vi "3 Phase Generator PMU Testing.vi"() -> ()   [LabVIEW 2022 SP3]
uses:
  <vilib>/Utility/TDMS File Viewer/NI_TDMS File Viewer.lvlib
  <vilib>/measure/NI_MAPro.lvlib
  <vilib>/Waveform/WDTOps.llb/WDT Get Waveform Time Array DBL.vi
  <vilib>/measure/maresamp.llb/Align 1 + N Waveforms (continuous).vi
panel:
  out "Phase 2":picture caption="Phasors visualization"
  in  "Data type":i32=8
  in  "ROCOF":dbl caption="Offset"
  in  "Data save 2":bool
  in  "Data save":bool
  in  "?":enum32{"Test set-up", "Set up"}(tab)
  out "h2rad":string="rad"
  out "h1rad":string="rad"
  out "h2deg\nH2deg":string="deg"
  out "H1deg":string="deg"
  out "H2V":string="V"
  out "H1V":string="V"
  out "H2pu":string="pu"
  out "H1pu":string="pu"
  out "PMrad":string="rad"
  out "PMdeg":string="deg"
  out "PMFeq":string="Hz"
  out "FreqDev":string="Hz"
  out "second":string="s"
  out "Hz/s":string="Hz/s"
  out "Final freq":string="Hz"
  out "Voltage step (V)":string="V"
  out "Voltage step (pu)":string="pu"
  out "?":string="Hz"
  out "AM (V)":string="V"
  out "AM (pu)":string="pu"
  out "?":string="Hz"
  out "?":string="Hz"
  out "?":string="V"
  out "?":string="pu"
  in  "H2 order":dbl=5.0 format="%#_13g"
  in  "Start":bool
  in  "Final freq.":dbl=55.0 format="%.2f"
  in  "ROCOF rate":dbl=1.0 format="%.2f"
  in  "Select test type":u16(ring) items=["Steady state", "Voltage step", "Phase step", "Frequency step", "Frequency ramp", "Amplitude modulation", "Phase modulation", "Harmonics"]
  in  "Frequency step":dbl caption="Offset" min=-5.0 max=5.0 format="%#.6f"
  in  "Phase step":dbl caption="Offset" min=-360.0 max=360.0 format="%#.6f"
  in  "Phase":dbl caption="Offset" min=-360.0 max=360.0
  in  "Voltage":dbl=1.0 caption="Offset" max=1.25 format="%#_5g"
  in  "Voltage step":dbl caption="Offset" min=-0.25 max=0.25 format="%#.6f"
  in  "Frequency":dbl=50.0 caption="Offset" max=55.0 format="%#_7g"
  in  "Mod Freq":dbl=1.0 caption="Offset" min=0.0 max=2.384 step=0.1 format="%#.6f"
  in  "Mod Amp":dbl=0.1 caption="Offset" max=0.125 format="%#.4f"
  in  "Mod Amp":dbl=0.1 caption="Offset" max=15.0 format="%#.4f"
  in  "Mod Freq":dbl=1.0 caption="Offset" format="%#.6f"
  in  "Nominal voltage":dbl=230.0 caption="Offset" format="%_6f"
  in  "stop":bool
  in  "Phase":dbl caption="Offset"
  in  "H1 Volt":dbl=0.05 format="%#_13g"
  in  "H2 Volt":dbl=0.05 format="%#_13g"
  in  "H1 Phase":dbl format="%#_13g"
  in  "H1 order":dbl=3.0 format="%#_13g"
  in  "H2 Phase":dbl format="%#_13g"
  out "Freq Dev":dbl caption="Offset" max=15.0 format="%#.4f"
  out "ROCOF":dbl
  out "Frequency":dbl=50.0 format="%#.8g"
  out "Voltage":dbl=1.0 format="%#_7g"
  out "Phase":dbl
  out "Phase (rad)":string="rad"
  out "Phase (deg)":string="deg"
  out "Time":dbl
  in  "File Name":string="testfile.tdms" caption="File name"
  in  "start":bool
  out "Phase step (rad)":string="rad"
  out "Phase step (deg)":string="deg"
  in  "Nominal Voltage":dbl=230.0 format="%#_13g"
  out "Transmitted Data":string
  in  "Voltage unit":u16(ring)=1 items=["Nominal voltage", "Per-unit voltage"]
  in  "Phase unit":u16(ring) items=["Degree", "Radian"]
  in  "Sampling info":cluster{"Fs":dbl, "#s":dbl}={"Fs"=10000.0, "#s"=1000.0} {"Fs" format="%.2p"}
  in  "LAN Module IP Address":string
  in  "LAN Port":u16
  in  "Nominal Frequency":dbl=50.0 format="%#_13g"
  out "Phase waveform 2":dbl(graph)
  in  "Initial freq.":dbl=50.0 format="%.2f"
  out "ROCOF waveform 2":dbl(graph)
  out "ROCOF waveform":dynamicdata(graph)
  out "Frequency waveform 2":dbl(graph)
  out "Frequency waveform":dynamicdata(graph)
  out "Votlage waveform":dynamicdata(graph)
  out "Numeric":i32
  out "resulting string 2":string
  out "double precision float":dbl[](array[numeric])
  out "Array 3":dbl[](array[numeric])
  out "Array 2":dbl[](array[numeric])
  out "Array":dbl[](array[numeric])
  out "Phase waveform":waveform(dbl)(graph)
  # "Current phasor values"
  # "UDP Protocol"
  # "Waveform scaling"
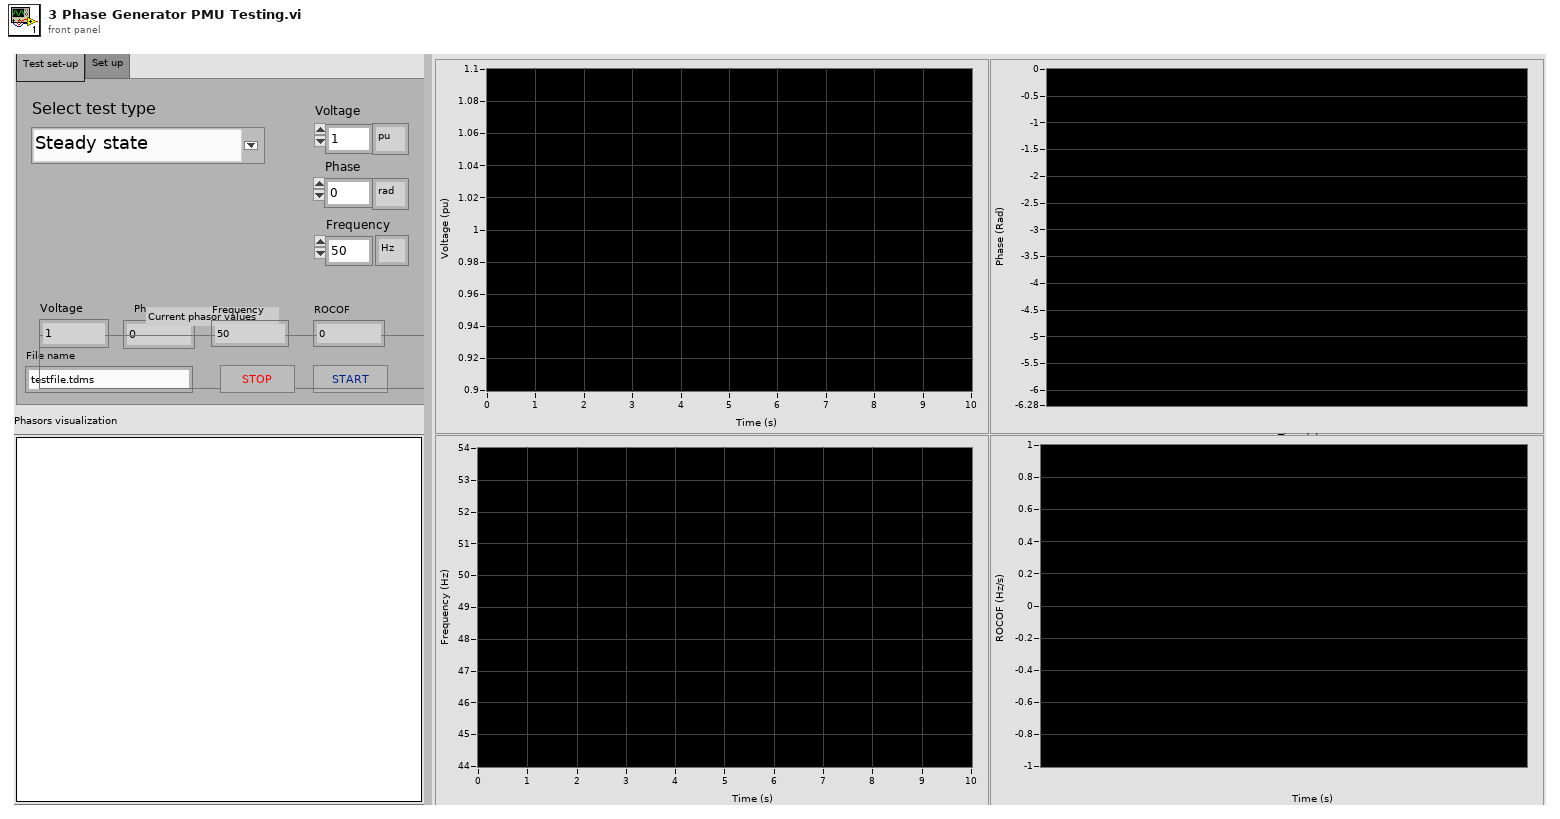
[diagram p1: front panel]
types:
  T1 = enum16{"open", "open or create", "create or replace", "create", "open (read-only)"}
  T2 = cluster{"maximum":dbl, "minimum":dbl, "clip to min":bool, "log?(F)":bool, "grid color":u32, "plot color":u32, "fmt and prec":cluster{"format":enum8{"Decimal", "Scientific", "Engineering", "Binary", "Octal", "Hex"}, "precision":u8}, "visible section":u16}
  T3 = typedef "LVBoundsTypeDef.ctl" = cluster{"Width":u32, "Height":u32}
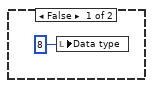
[diagram p2: hidden frame]
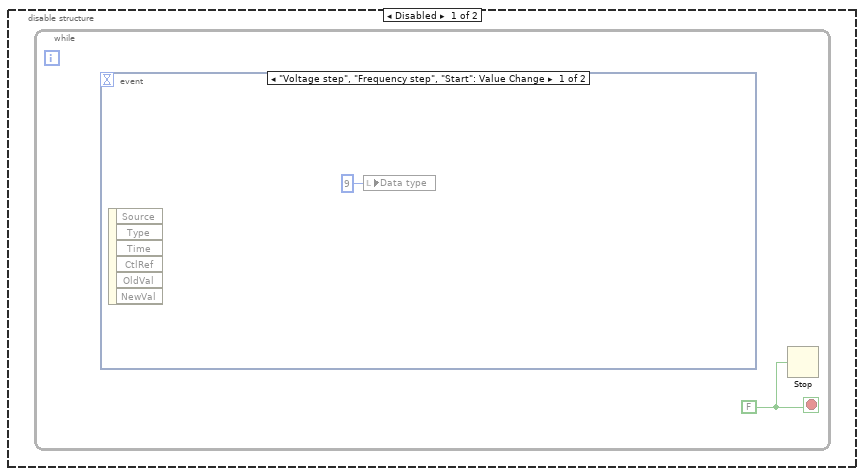
[diagram p3: hidden frame]
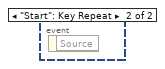
[diagram p4: hidden frame]
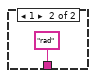
[diagram p5: hidden frame]
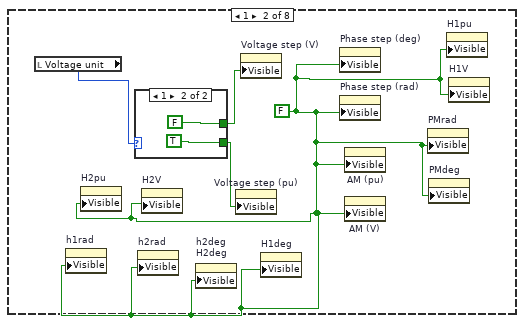
[diagram p6: hidden frame]
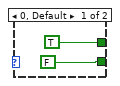
[diagram p7: hidden frame]
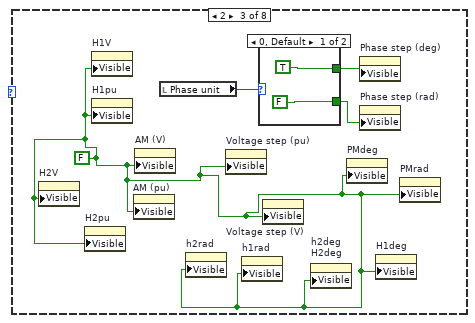
[diagram p8: hidden frame]
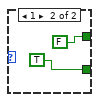
[diagram p9: hidden frame]
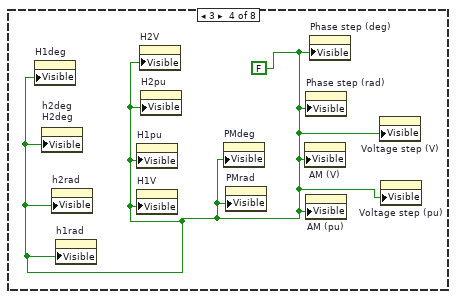
[diagram p10: hidden frame]
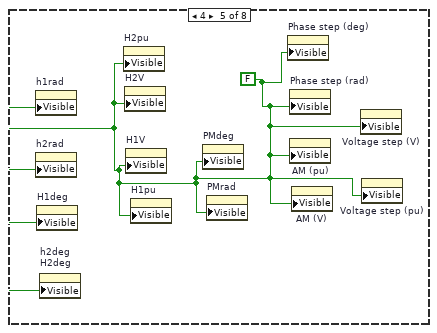
[diagram p11: hidden frame]
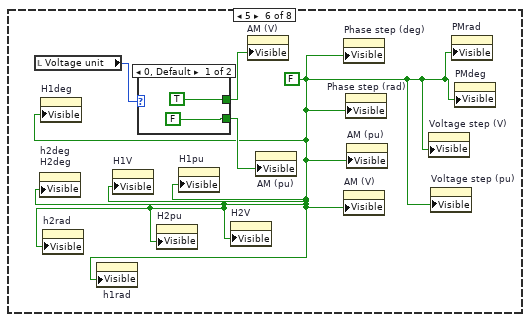
[diagram p12: hidden frame]
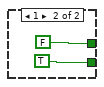
[diagram p13: hidden frame]
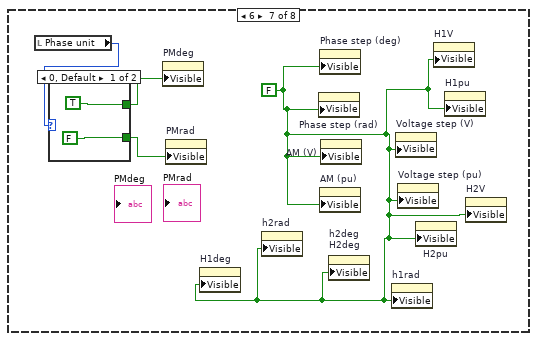
[diagram p14: hidden frame]
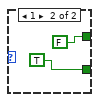
[diagram p15: hidden frame]
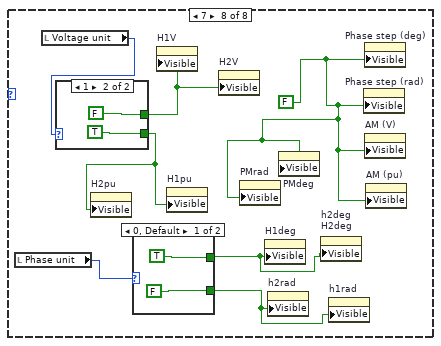
[diagram p16: hidden frame]
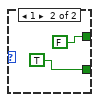
[diagram p17: hidden frame]
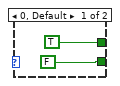
[diagram p18: hidden frame]
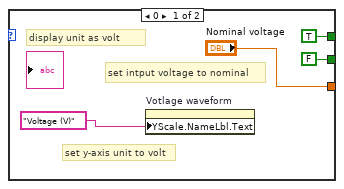
[diagram p19: hidden frame]
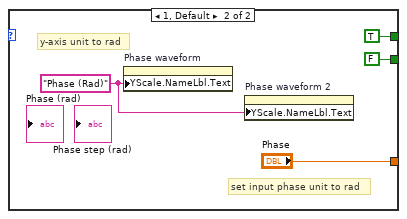
[diagram p20: hidden frame]
diagram:
  n1 = call <vilib>:"Application Directory.vi"() -> ("Application Directory"=w5:path)
  n2 = Concatenate Strings("measurements\\", "File Name") -> (w3:string)
  n3 = Build Path(base path=w5, name or relative path=w3) -> (appended path=w4:path)
  n4 = flat-sequence {
    frame #0 {
      w23 = FALSE
      n5 = local read "Data type"() -> (w29:i32)
      n6 = local read "start"() -> (w22:bool)
      n7 = Equal?(x=w29, y=8) -> (x = y?=w28:bool)
      n8 = Equal?(x=w22, y=TRUE) -> (x = y?=w27:bool)
      n9 = And(x=w27, y=w28) -> (x .and. y?=w26:bool)
      n10 = case shown="True" w26 {
        frame False {
          n11 = local write "Data type"(8 ("Data type")) -> ()
        }
        frame True {
          n12 = local write "Data type"(9 ("Data type")) -> ()
        }
      }
      n13 = property on="Start" class="Bool (strict)"("Value"=w23) -> ()  [unwired: 2 in, 2 out]
      n14 = property on="start" class="Bool (strict)"("Value"=w23) -> ()  [unwired: 2 in, 2 out]
    }
  }
  n15 = TDMS Open(10:T1."create or replace" ("operation (0:open)"), 11:w4) -> (0:w14:errorcluster, 3:w15:refnum<k34>)  [unwired: 5 in]
  n16 = TDMS Set Properties(5:"Data file for PMU testing", 7:"title", 8:w14, 11:w15) -> (0:w12:errorcluster, 3:w13:refnum<k34>)  [unwired: 2 in, 2 out]
  n17 = Get Date/Time In Seconds() -> (seconds since 1Jan1904=w16:timestamp)
  n18 = TDMS Set Properties(5:w16, 7:"datetime", 8:w12, 11:w13) -> (0:w7:errorcluster, 3:w6:refnum<k34>)  [unwired: 2 in, 2 out]
  n19 = while {
    tunnel: [w37] -> w18
    tunnel: [w36] -> w17
    tunnel: w7 -> [w34]
    tunnel: w6 -> [w35]
    i -> [w69]
    stop <- "stop" stop-if-true
    w44 = "3 Phase Generator" ("group name in (Untitled)")
    # "amplitude modulation\nmod freq unit"
    # "phase \nmodulation\namplitude \nunit"
    # "stop button"
    # "box for config layout"
    n20 = flat-sequence {
      tunnel: ["start"] -> w40
      tunnel: ["start"] -> _
      tunnel: [w87] -> w43
      tunnel: [w82] -> w42
      tunnel: [w85] -> w41
      tunnel: w40 -> [w87]
      tunnel: [w166] -> w74
      tunnel: w43 -> [w166]
      tunnel: w42 -> [w160]
      tunnel: w41 -> [w178]
      tunnel: w39 -> [w174]
      tunnel: w38 -> [w173]
      tunnel: [w172] -> w37
      tunnel: [w171] -> w36
      tunnel: w74 -> [w790]
      frame #0 {
        # "input freq unit"
        # "start button"
      }
      frame #1 {
        # "voltage step"
        # "amplitude modulation unit"
        # "set default angle unit ot rad\nif input deg, convert to rad"
        # "enable nominal voltage"
        # "enable unit volt"
        # "enable unit per-unit"
        # "enable per-unit voltage"
        # "per-unit voltage or nominal voltage"
        n21 = local read "Select test type"() -> (w80:u16)
        n22 = case shown="0" "Phase unit" {
          tunnel: [w147 "Phase"] -> w82
          tunnel: [FALSE TRUE] -> w78
          tunnel: [TRUE FALSE] -> w79
          frame 0 {
            # "convert deg to rad"
            # "y-axis in deg"
            # "set inputphase unit to deg"
            n23 = property on="Phase waveform" class="WFChart (strict)"("YScale.NameLbl.Text"="Phase (deg)" ("Y Scale.Name Label.Text")) -> ()  [unwired: 2 in, 2 out]
            n24 = Multiply(x="Phase", y=3.141592653589793) -> (x*y=w150:dbl)
            n25 = Divide(x=w150, y=180.0) -> (x/y=w147:dbl)
          }
          frame 1, Default {
            w154 = "Phase (Rad)" ("Y Scale.Name Label.Text")
            # "y-axis unit to rad"
            # "set input phase unit to rad"
            n26 = property on="Phase waveform" class="WFChart (strict)"("YScale.NameLbl.Text"=w154) -> ()  [unwired: 2 in, 2 out]
            n27 = property on="Phase waveform 2" class="WFChart (strict)"("YScale.NameLbl.Text"=w154) -> ()  [unwired: 2 in, 2 out]
          }
        }
        n28 = case shown="0, Default" w80 {
          frame 0, Default {
            w88 = FALSE
            n29 = property on="H2V" class="Str"("Visible"=w88) -> ()  [unwired: 2 in, 2 out]
            n30 = property on="H2pu" class="Str"("Visible"=w88) -> ()  [unwired: 2 in, 2 out]
            n31 = property on="h1rad" class="Str"("Visible"=w88) -> ()  [unwired: 2 in, 2 out]
            n32 = property on="H1deg" class="Str"("Visible"=w88) -> ()  [unwired: 2 in, 2 out]
            n33 = property on="H1V" class="Str"("Visible"=w88) -> ()  [unwired: 2 in, 2 out]
            n34 = property on="H1pu" class="Str"("Visible"=w88) -> ()  [unwired: 2 in, 2 out]
            n35 = property on="h2rad" class="Str"("Visible"=w88) -> ()  [unwired: 2 in, 2 out]
            n36 = property on="h2deg\nH2deg" class="Str"("Visible"=w88) -> ()  [unwired: 2 in, 2 out]
            n37 = property on="PMdeg" class="Str"("Visible"=w88) -> ()  [unwired: 2 in, 2 out]
            n38 = property on="PMrad" class="Str"("Visible"=w88) -> ()  [unwired: 2 in, 2 out]
            n39 = property on="Voltage step (pu)" class="Str"("Visible"=w88) -> ()  [unwired: 2 in, 2 out]
            n40 = property on="AM (pu)" class="Str"("Visible"=w88) -> ()  [unwired: 2 in, 2 out]
            n41 = property on="AM (V)" class="Str"("Visible"=w88) -> ()  [unwired: 2 in, 2 out]
            n42 = property on="Phase step (deg)" class="Str"("Visible"=w88) -> ()  [unwired: 2 in, 2 out]
            n43 = property on="Phase step (rad)" class="Str"("Visible"=w88) -> ()  [unwired: 2 in, 2 out]
            n44 = property on="Voltage step (V)" class="Str"("Visible"=w88) -> ()  [unwired: 2 in, 2 out]
          }
          frame 1 {
            w89 = FALSE
            n45 = local read "Voltage unit"() -> (w92:u16)
            n46 = property on="h1rad" class="Str"("Visible"=w89) -> ()  [unwired: 2 in, 2 out]
            n47 = property on="H2pu" class="Str"("Visible"=w89) -> ()  [unwired: 2 in, 2 out]
            n48 = case shown="1" w92 {
              tunnel: [TRUE FALSE] -> w90
              tunnel: [FALSE TRUE] -> w91
              frame 0, Default {
              }
              frame 1 {
              }
            }
            n49 = property on="h2rad" class="Str"("Visible"=w89) -> ()  [unwired: 2 in, 2 out]
            n50 = property on="H2V" class="Str"("Visible"=w89) -> ()  [unwired: 2 in, 2 out]
            n51 = property on="h2deg\nH2deg" class="Str"("Visible"=w89) -> ()  [unwired: 2 in, 2 out]
            n52 = property on="Voltage step (pu)" class="Str"("Visible"=w91) -> ()  [unwired: 2 in, 2 out]
            n53 = property on="Voltage step (V)" class="Str"("Visible"=w90) -> ()  [unwired: 2 in, 2 out]
            n54 = property on="H1deg" class="Str"("Visible"=w89) -> ()  [unwired: 2 in, 2 out]
            n55 = property on="Phase step (deg)" class="Str"("Visible"=w89) -> ()  [unwired: 2 in, 2 out]
            n56 = property on="Phase step (rad)" class="Str"("Visible"=w89) -> ()  [unwired: 2 in, 2 out]
            n57 = property on="AM (pu)" class="Str"("Visible"=w89) -> ()  [unwired: 2 in, 2 out]
            n58 = property on="AM (V)" class="Str"("Visible"=w89) -> ()  [unwired: 2 in, 2 out]
            n59 = property on="PMrad" class="Str"("Visible"=w89) -> ()  [unwired: 2 in, 2 out]
            n60 = property on="PMdeg" class="Str"("Visible"=w89) -> ()  [unwired: 2 in, 2 out]
            n61 = property on="H1pu" class="Str"("Visible"=w89) -> ()  [unwired: 2 in, 2 out]
            n62 = property on="H1V" class="Str"("Visible"=w89) -> ()  [unwired: 2 in, 2 out]
          }
          frame 2 {
            w97 = FALSE
            n63 = property on="H2V" class="Str"("Visible"=w97) -> ()  [unwired: 2 in, 2 out]
            n64 = property on="H2pu" class="Str"("Visible"=w97) -> ()  [unwired: 2 in, 2 out]
            n65 = property on="H1V" class="Str"("Visible"=w97) -> ()  [unwired: 2 in, 2 out]
            n66 = property on="H1pu" class="Str"("Visible"=w97) -> ()  [unwired: 2 in, 2 out]
            n67 = property on="AM (pu)" class="Str"("Visible"=w97) -> ()  [unwired: 2 in, 2 out]
            n68 = property on="AM (V)" class="Str"("Visible"=w97) -> ()  [unwired: 2 in, 2 out]
            n69 = local read "Phase unit"() -> (w98:u16)
            n70 = property on="h2rad" class="Str"("Visible"=w97) -> ()  [unwired: 2 in, 2 out]
            n71 = property on="Voltage step (pu)" class="Str"("Visible"=w97) -> ()  [unwired: 2 in, 2 out]
            n72 = property on="h1rad" class="Str"("Visible"=w97) -> ()  [unwired: 2 in, 2 out]
            n73 = case shown="0, Default" w98 {
              tunnel: [TRUE FALSE] -> w100
              tunnel: [FALSE TRUE] -> w99
              frame 0, Default {
              }
              frame 1 {
              }
            }
            n74 = property on="Voltage step (V)" class="Str"("Visible"=w97) -> ()  [unwired: 2 in, 2 out]
            n75 = property on="h2deg\nH2deg" class="Str"("Visible"=w97) -> ()  [unwired: 2 in, 2 out]
            n76 = property on="PMdeg" class="Str"("Visible"=w97) -> ()  [unwired: 2 in, 2 out]
            n77 = property on="Phase step (deg)" class="Str"("Visible"=w100) -> ()  [unwired: 2 in, 2 out]
            n78 = property on="Phase step (rad)" class="Str"("Visible"=w99) -> ()  [unwired: 2 in, 2 out]
            n79 = property on="H1deg" class="Str"("Visible"=w97) -> ()  [unwired: 2 in, 2 out]
            n80 = property on="PMrad" class="Str"("Visible"=w97) -> ()  [unwired: 2 in, 2 out]
          }
          frame 3 {
            w105 = FALSE
            n81 = property on="H1deg" class="Str"("Visible"=w105) -> ()  [unwired: 2 in, 2 out]
            n82 = property on="h2deg\nH2deg" class="Str"("Visible"=w105) -> ()  [unwired: 2 in, 2 out]
            n83 = property on="h2rad" class="Str"("Visible"=w105) -> ()  [unwired: 2 in, 2 out]
            n84 = property on="h1rad" class="Str"("Visible"=w105) -> ()  [unwired: 2 in, 2 out]
            n85 = property on="H1pu" class="Str"("Visible"=w105) -> ()  [unwired: 2 in, 2 out]
            n86 = property on="H1V" class="Str"("Visible"=w105) -> ()  [unwired: 2 in, 2 out]
            n87 = property on="H2V" class="Str"("Visible"=w105) -> ()  [unwired: 2 in, 2 out]
            n88 = property on="H2pu" class="Str"("Visible"=w105) -> ()  [unwired: 2 in, 2 out]
            n89 = property on="PMdeg" class="Str"("Visible"=w105) -> ()  [unwired: 2 in, 2 out]
            n90 = property on="PMrad" class="Str"("Visible"=w105) -> ()  [unwired: 2 in, 2 out]
            n91 = property on="AM (V)" class="Str"("Visible"=w105) -> ()  [unwired: 2 in, 2 out]
            n92 = property on="Phase step (rad)" class="Str"("Visible"=w105) -> ()  [unwired: 2 in, 2 out]
            n93 = property on="AM (pu)" class="Str"("Visible"=w105) -> ()  [unwired: 2 in, 2 out]
            n94 = property on="Phase step (deg)" class="Str"("Visible"=w105) -> ()  [unwired: 2 in, 2 out]
            n95 = property on="Voltage step (V)" class="Str"("Visible"=w105) -> ()  [unwired: 2 in, 2 out]
            n96 = property on="Voltage step (pu)" class="Str"("Visible"=w105) -> ()  [unwired: 2 in, 2 out]
          }
          frame 4 {
            w106 = FALSE
            n97 = property on="h1rad" class="Str"("Visible"=w106) -> ()  [unwired: 2 in, 2 out]
            n98 = property on="h2rad" class="Str"("Visible"=w106) -> ()  [unwired: 2 in, 2 out]
            n99 = property on="H1deg" class="Str"("Visible"=w106) -> ()  [unwired: 2 in, 2 out]
            n100 = property on="h2deg\nH2deg" class="Str"("Visible"=w106) -> ()  [unwired: 2 in, 2 out]
            n101 = property on="H2pu" class="Str"("Visible"=w106) -> ()  [unwired: 2 in, 2 out]
            n102 = property on="H2V" class="Str"("Visible"=w106) -> ()  [unwired: 2 in, 2 out]
            n103 = property on="H1V" class="Str"("Visible"=w106) -> ()  [unwired: 2 in, 2 out]
            n104 = property on="H1pu" class="Str"("Visible"=w106) -> ()  [unwired: 2 in, 2 out]
            n105 = property on="PMdeg" class="Str"("Visible"=w106) -> ()  [unwired: 2 in, 2 out]
            n106 = property on="PMrad" class="Str"("Visible"=w106) -> ()  [unwired: 2 in, 2 out]
            n107 = property on="Phase step (deg)" class="Str"("Visible"=w106) -> ()  [unwired: 2 in, 2 out]
            n108 = property on="Phase step (rad)" class="Str"("Visible"=w106) -> ()  [unwired: 2 in, 2 out]
            n109 = property on="AM (pu)" class="Str"("Visible"=w106) -> ()  [unwired: 2 in, 2 out]
            n110 = property on="AM (V)" class="Str"("Visible"=w106) -> ()  [unwired: 2 in, 2 out]
            n111 = property on="Voltage step (V)" class="Str"("Visible"=w106) -> ()  [unwired: 2 in, 2 out]
            n112 = property on="Voltage step (pu)" class="Str"("Visible"=w106) -> ()  [unwired: 2 in, 2 out]
          }
          frame 5 {
            w107 = FALSE
            n113 = local read "Voltage unit"() -> (w110:u16)
            n114 = property on="h2deg\nH2deg" class="Str"("Visible"=w107) -> ()  [unwired: 2 in, 2 out]
            n115 = property on="H1deg" class="Str"("Visible"=w107) -> ()  [unwired: 2 in, 2 out]
            n116 = property on="h2rad" class="Str"("Visible"=w107) -> ()  [unwired: 2 in, 2 out]
            n117 = property on="h1rad" class="Str"("Visible"=w107) -> ()  [unwired: 2 in, 2 out]
            n118 = property on="H1V" class="Str"("Visible"=w107) -> ()  [unwired: 2 in, 2 out]
            n119 = case shown="0, Default" w110 {
              tunnel: [TRUE FALSE] -> w109
              tunnel: [FALSE TRUE] -> w108
              frame 0, Default {
              }
              frame 1 {
              }
            }
            n120 = property on="H2pu" class="Str"("Visible"=w107) -> ()  [unwired: 2 in, 2 out]
            n121 = property on="H1pu" class="Str"("Visible"=w107) -> ()  [unwired: 2 in, 2 out]
            n122 = property on="H2V" class="Str"("Visible"=w107) -> ()  [unwired: 2 in, 2 out]
            n123 = property on="AM (V)" class="Str"("Visible"=w109) -> ()  [unwired: 2 in, 2 out]
            n124 = property on="AM (pu)" class="Str"("Visible"=w108) -> ()  [unwired: 2 in, 2 out]
            n125 = property on="Phase step (deg)" class="Str"("Visible"=w107) -> ()  [unwired: 2 in, 2 out]
            n126 = property on="AM (V)" class="Str"("Visible"=w107) -> ()  [unwired: 2 in, 2 out]
            n127 = property on="Phase step (rad)" class="Str"("Visible"=w107) -> ()  [unwired: 2 in, 2 out]
            n128 = property on="AM (pu)" class="Str"("Visible"=w107) -> ()  [unwired: 2 in, 2 out]
            n129 = property on="Voltage step (V)" class="Str"("Visible"=w107) -> ()  [unwired: 2 in, 2 out]
            n130 = property on="Voltage step (pu)" class="Str"("Visible"=w107) -> ()  [unwired: 2 in, 2 out]
            n131 = property on="PMrad" class="Str"("Visible"=w107) -> ()  [unwired: 2 in, 2 out]
            n132 = property on="PMdeg" class="Str"("Visible"=w107) -> ()  [unwired: 2 in, 2 out]
          }
          frame 6 {
            w115 = FALSE
            n133 = local read "Phase unit"() -> (w118:u16)
            n134 = case shown="0, Default" w118 {
              tunnel: [TRUE FALSE] -> w117
              tunnel: [FALSE TRUE] -> w116
              frame 0, Default {
              }
              frame 1 {
              }
            }
            n135 = property on="PMdeg" class="Str"("Visible"=w117) -> ()  [unwired: 2 in, 2 out]
            n136 = property on="PMrad" class="Str"("Visible"=w116) -> ()  [unwired: 2 in, 2 out]
            n137 = property on="H1deg" class="Str"("Visible"=w115) -> ()  [unwired: 2 in, 2 out]
            n138 = property on="h2rad" class="Str"("Visible"=w115) -> ()  [unwired: 2 in, 2 out]
            n139 = property on="Phase step (rad)" class="Str"("Visible"=w115) -> ()  [unwired: 2 in, 2 out]
            n140 = property on="Phase step (deg)" class="Str"("Visible"=w115) -> ()  [unwired: 2 in, 2 out]
            n141 = property on="AM (pu)" class="Str"("Visible"=w115) -> ()  [unwired: 2 in, 2 out]
            n142 = property on="AM (V)" class="Str"("Visible"=w115) -> ()  [unwired: 2 in, 2 out]
            n143 = property on="h2deg\nH2deg" class="Str"("Visible"=w115) -> ()  [unwired: 2 in, 2 out]
            n144 = property on="h1rad" class="Str"("Visible"=w115) -> ()  [unwired: 2 in, 2 out]
            n145 = property on="Voltage step (V)" class="Str"("Visible"=w115) -> ()  [unwired: 2 in, 2 out]
            n146 = property on="Voltage step (pu)" class="Str"("Visible"=w115) -> ()  [unwired: 2 in, 2 out]
            n147 = property on="H2pu" class="Str"("Visible"=w115) -> ()  [unwired: 2 in, 2 out]
            n148 = property on="H1V" class="Str"("Visible"=w115) -> ()  [unwired: 2 in, 2 out]
            n149 = property on="H1pu" class="Str"("Visible"=w115) -> ()  [unwired: 2 in, 2 out]
            n150 = property on="H2V" class="Str"("Visible"=w115) -> ()  [unwired: 2 in, 2 out]
          }
          frame 7 {
            w129 = FALSE
            n151 = local read "Phase unit"() -> (w123:u16)
            n152 = local read "Voltage unit"() -> (w128:u16)
            n153 = case shown="1" w128 {
              tunnel: [TRUE FALSE] -> w127
              tunnel: [FALSE TRUE] -> w126
              frame 0, Default {
              }
              frame 1 {
              }
            }
            n154 = property on="H2pu" class="Str"("Visible"=w126) -> ()  [unwired: 2 in, 2 out]
            n155 = case shown="0, Default" w123 {
              tunnel: [TRUE FALSE] -> w125
              tunnel: [FALSE TRUE] -> w124
              frame 0, Default {
              }
              frame 1 {
              }
            }
            n156 = property on="H1V" class="Str"("Visible"=w127) -> ()  [unwired: 2 in, 2 out]
            n157 = property on="H1pu" class="Str"("Visible"=w126) -> ()  [unwired: 2 in, 2 out]
            n158 = property on="H2V" class="Str"("Visible"=w127) -> ()  [unwired: 2 in, 2 out]
            n159 = property on="PMrad" class="Str"("Visible"=w129) -> ()  [unwired: 2 in, 2 out]
            n160 = property on="H1deg" class="Str"("Visible"=w125) -> ()  [unwired: 2 in, 2 out]
            n161 = property on="h2rad" class="Str"("Visible"=w124) -> ()  [unwired: 2 in, 2 out]
            n162 = property on="PMdeg" class="Str"("Visible"=w129) -> ()  [unwired: 2 in, 2 out]
            n163 = property on="h2deg\nH2deg" class="Str"("Visible"=w125) -> ()  [unwired: 2 in, 2 out]
            n164 = property on="h1rad" class="Str"("Visible"=w124) -> ()  [unwired: 2 in, 2 out]
            n165 = property on="Phase step (rad)" class="Str"("Visible"=w129) -> ()  [unwired: 2 in, 2 out]
            n166 = property on="Phase step (deg)" class="Str"("Visible"=w129) -> ()  [unwired: 2 in, 2 out]
            n167 = property on="AM (V)" class="Str"("Visible"=w129) -> ()  [unwired: 2 in, 2 out]
            n168 = property on="AM (pu)" class="Str"("Visible"=w129) -> ()  [unwired: 2 in, 2 out]
          }
        }
        n169 = case shown="1, Default" "Voltage unit" {
          tunnel: ["Nominal voltage" "Voltage"] -> w85
          tunnel: [TRUE FALSE] -> w83
          tunnel: [FALSE TRUE] -> w84
          frame 0 {
            # "set intput voltage to nominal"
            # "display unit as volt"
            # "set y-axis unit to volt"
            n170 = property on="Votlage waveform" class="WFChart (strict)"("YScale.NameLbl.Text"="Voltage (V)" ("Y Scale.Name Label.Text")) -> ()  [unwired: 2 in, 2 out]
          }
          frame 1, Default {
            # "set voltage unit to pu"
            # "set y-axis to show in per-unit scale"
            n171 = property on="Votlage waveform" class="WFChart (strict)"("YScale.NameLbl.Text"="Voltage (pu)" ("Y Scale.Name Label.Text")) -> ()  [unwired: 2 in, 2 out]
          }
        }
        n172 = property on="AM (pu)" class="Str" props=["Visible"]() -> ()  [unwired: 2 in, 3 out]
        n173 = property on="AM (pu)" class="Str" props=["Visible"]() -> ()  [unwired: 2 in, 3 out]
        n174 = property on="Phase (deg)" class="Str"("Visible"=w79) -> ()  [unwired: 2 in, 2 out]
        n175 = property on="Phase (rad)" class="Str"("Visible"=w78) -> ()  [unwired: 2 in, 2 out]
        n176 = property class="Str"("Visible"=w84) -> ()  [unwired: 2 in, 2 out]
        n177 = property on="Nominal voltage" class="DigNum (strict)"("Visible"=w83) -> ()  [unwired: 2 in, 2 out]
        n178 = property class="Str"("Visible"=w83) -> ()  [unwired: 2 in, 2 out]
        n179 = property on="Voltage" class="DigNum (strict)"("Visible"=w84) -> ()  [unwired: 2 in, 2 out]
        n180 = property on="Phase (rad)" class="DigNum (strict)"("Visible"=w78) -> ()  [unwired: 2 in, 2 out]
        n181 = property on="Phase (deg)" class="DigNum (strict)"("Visible"=w79) -> ()  [unwired: 2 in, 2 out]
        n182 = invoke on="double precision float" class="Arr (strict)" method="Reinit To Default"() -> ()  [unwired: 3 in, 3 out]
      }
      frame #2 {
        # "phase in"
        # "voltage in"
        # "start generating"
        n183 = invoke on="Array 3" class="Arr (strict)" method="Reinit To Default"() -> ()  [unwired: 3 in, 3 out]
        n184 = invoke on="Array 2" class="Arr (strict)" method="Reinit To Default"() -> ()  [unwired: 3 in, 3 out]
        n185 = invoke on="Array" class="Arr (strict)" method="Reinit To Default"() -> ()  [unwired: 3 in, 3 out]
        n186 = case shown="True" w166 {
          selector: w166 -> [_ w254]
          tunnel: "Select test type" -> [w224 w262]
          tunnel: [w220 w259] -> w163
          tunnel: [w223 w250] -> w176
          tunnel: [w218 w247] -> _
          tunnel: [w217 w251] -> w158
          tunnel: [w215 w248] -> w164
          tunnel: [w219 w249] -> w165
          tunnel: [w216 w258] -> w159
          tunnel: [w221 w257] -> _
          tunnel: [w222 w256] -> w162
          tunnel: [w209 w255] -> w161
          tunnel: w160 -> [_ w253]
          tunnel: w178 -> [_ w252]
          tunnel: [w214 w246] -> w177
          tunnel: [w213 w245] -> w175
          tunnel: [w212 w244] -> w170
          tunnel: [w212 w243] -> w169
          tunnel: [w212 w242] -> w168
          tunnel: [w212 w241] -> w167
          frame False {
            w210 = dbl[] [] ("History Data")
            w212 = dbl[] []
            w211 = waveform(dbl)[] [] ("History Data")
            n187 = property on="Frequency waveform 2" class="WFChart (strict)"("History Data"=w210) -> ()  [unwired: 2 in, 2 out]
            n188 = property on="ROCOF waveform 2" class="WFChart (strict)"("History Data"=w210) -> ()  [unwired: 2 in, 2 out]
            n189 = property on="Phase waveform 2" class="WFChart (strict)"("History Data"=w210) -> ()  [unwired: 2 in, 2 out]
            n190 = property on="Frequency waveform" class="WFChart (strict)"("History Data"=w211) -> ()  [unwired: 2 in, 2 out]
            n191 = property on="Phase waveform" class="WFChart (strict)"("History Data"=w211) -> ()  [unwired: 2 in, 2 out]
            n192 = property on="Votlage waveform" class="WFChart (strict)"("History Data"=w211) -> ()  [unwired: 2 in, 2 out]
            n193 = property on="ROCOF waveform" class="WFChart (strict)"("History Data"=w211) -> ()  [unwired: 2 in, 2 out]
            n194 = case shown="0, Default" w224 {
              tunnel: [w226 w228 w229 w231 w234 w236 w238 w239] -> _
              tunnel: [w226 w228 w229 w231 w234 w236 w238 w240] -> w223
              tunnel: [w225 w227 w230 w232 w233 w236 w237 w239] -> w222
              tunnel: [w225 w227 w230 w232 w233 w235 w238 w239] -> w209
              tunnel: [w225 w227 w230 w232 w233 w235 w237 w239] -> w221
              tunnel: [w225 w227 w229 w232 w233 w235 w237 w239] -> w220
              tunnel: [w225 w227 w230 w231 w233 w235 w237 w239] -> w219
              tunnel: [w225 w227 w230 w232 w233 w235 w237 w239] -> w218
              tunnel: [w225 w227 w230 w232 w233 w235 w237 w240] -> w215
              tunnel: [w225 w228 w230 w232 w233 w235 w237 w239] -> w217
              tunnel: [w225 w227 w230 w232 w234 w235 w237 w239] -> w216
              tunnel: [w225 w227 w229 w232 w233 w235 w237 w239] -> w214
              tunnel: [w225 w227 w229 w231 w233 w235 w237 w239] -> w213
              frame 0, Default {
                w226 = TRUE
                w225 = FALSE
              }
              frame 1 {
                w228 = TRUE
                w227 = FALSE
              }
              frame 2 {
                w229 = TRUE
                w230 = FALSE
              }
              frame 3 {
                w231 = TRUE
                w232 = FALSE
              }
              frame 4 {
                w234 = TRUE
                w233 = FALSE
              }
              frame 5 {
                w236 = TRUE
                w235 = FALSE
              }
              frame 6 {
                w238 = TRUE
                w237 = FALSE
              }
              frame 7 {
                w239 = FALSE
                w240 = TRUE
              }
            }
          }
          frame True {
            # "phase mod freq dev unit"
            # "phase mod freq unit"
            n195 = case shown="0, Default" w262 {
              tunnel: w252 -> [w320 w367 w432 w499 w602 w688 w759 w787]
              tunnel: w253 -> [w263 w366 w430 w508 w615 w703 w734 _]
              tunnel: "Frequency" -> [w318 w362 w414 w513 w597 w700 w735 w789]
              tunnel: "ROCOF" -> [w313 w372 w410 w492 _ w699 w733 _]
              tunnel: [w294 w382 w421 w498 w631 w711 w765 w786] -> _
              tunnel: [w312 w357 w421 w501 w598 w686 w732 w786] -> w259
              tunnel: [w294 w382 w421 w498 w631 w711 w765 w788] -> w250
              tunnel: [w312 w357 w421 w501 w598 w711 w765 w788] -> w247
              tunnel: [w294 w382 w421 w498 w631 w711 w765 w786] -> _
              tunnel: [w312 w357 w444 w501 w598 w686 w732 w788] -> w248
              tunnel: [w312 w357 w444 w498 w598 w686 w732 w786] -> w249
              tunnel: [w312 w357 w444 w501 w631 w686 w732 w786] -> w258
              tunnel: [w312 w357 w444 w501 w598 w686 w732 w786] -> w257
              tunnel: [w312 w357 w444 w501 w598 w711 w732 w786] -> w256
              tunnel: [w312 w357 w444 w501 w598 w686 w765 w786] -> w255
              tunnel: w254 -> [_ _ _ _ _ _ _ _]
              tunnel: [w312 w382 w444 w501 w598 w686 w732 w786] -> w251
              tunnel: [w312 w357 w421 w501 w598 w686 w732 w786] -> w246
              tunnel: [w294 w357 w421 w498 w598 w686 w732 w786] -> w245
              tunnel: [w305 w354 w417 w487 w591 w682 w728 w785] -> w244
              tunnel: [w308 w355 w415 w496 w596 w681 w725 w785] -> w243
              tunnel: [w304 w353 w416 w488 w594 w684 w726 w785] -> w242
              tunnel: [w292 w356 w418 w495 w580 w683 w727 w785] -> w241
              frame 0, Default {
                w294 = TRUE
                w312 = FALSE
                # "initial phase"
                # "delta rocof = differenciate delta freq"
                # "delta phase = integrate delta freq"
                # "rocof func: f(t)=rocof"
                # "input freq: f(t)=f_in"
                # "voltage in func: f(t)=v_in"
                # "Steady state"
                n196 = local read "Sampling info"() -> (w300:cluster{"Fs":dbl, "#s":dbl})
                n197 = call <vilib>:"Formula Waveform.vi"("sampling info"=w300, "formula"="a", "amplitude"=w318) -> ("signal out"=w304:waveform(dbl))  [unwired: 7 in, 1 out]
                n198 = call <vilib>:"Formula Waveform.vi"("sampling info"=w300, "formula"="a", "amplitude"=w313) -> ("signal out"=w311:waveform(dbl))  [unwired: 7 in, 1 out]
                n199 = call "Sample Compression8"("Signals"=w304) -> ("Maximum"=w314:dynamicdata)  [unwired: 8 in, 2 out]
                "Frequency waveform" <- w314
                n200 = call <vilib>:"Formula Waveform.vi"("formula"="a", "amplitude"=w263) -> ("signal out"=w264:waveform(dbl))  [unwired: 8 in, 1 out]
                n201 = call <vilib>:"Formula Waveform.vi"("sampling info"=w300, "formula"="a", "amplitude"=w320) -> ("signal out"=w308:waveform(dbl))  [unwired: 7 in, 1 out]
                n202 = call <vilib>:"Formula Waveform.vi"("sampling info"=w300, "formula"="a", "amplitude"="Nominal Frequency") -> ("signal out"=w303:waveform(dbl))  [unwired: 7 in, 1 out]
                n203 = local write "Frequency"(w314) -> ()
                n204 = local read "Phase unit"() -> (w287:u16)
                n205 = Subtract(1:w303, 2:w304) -> (0:w272:waveform(dbl))  [unwired: 1 in, 1 out]
                n206 = call "Sample Compression6"("Signals"=w308) -> ("Maximum"=w315:dynamicdata)  [unwired: 8 in, 2 out]
                "Votlage waveform" <- w315
                n207 = case shown="0, Default" w287 {
                  tunnel: [360.0 6.283185307179586] -> w286
                  frame 0, Default {
                  }
                  frame 1 {
                  }
                }
                n208 = call "Integral (Sum[Xdt])2"("Signals"=w272) -> ("Result"=w271:dynamicdata)  [unwired: 5 in, 1 out]
                n209 = local write "Voltage"(w315) -> ()
                n210 = call <vilib>:"Formula Waveform.vi"("sampling info"=w300, "formula"="a", "amplitude"=w286) -> ("signal out"=w302:waveform(dbl))  [unwired: 7 in, 1 out]
                n211 = Multiply(x=6.283185307179586, y=w271) -> (x*y=w269:dynamicdata)
                n212 = call-poly <vilib>:"Align Waveforms (continuous).vi"("waveforms in"=w269, "waveform in"=w264) -> ("aligned waveforms out"=w266:waveform(dbl)[], "aligned waveform out"=w268:waveform(dbl))  [unwired: 7 in, 1 out]
                n213 = call "Sample Compression49"("Signals"=w302) -> ("Maximum"=w280:dynamicdata)  [unwired: 8 in, 2 out]
                n214 = call "Sample Compression35"("Signals"=w266) -> ("Maximum"=w265:dynamicdata)  [unwired: 8 in, 2 out]
                n215 = call "Sample Compression7"("Signals"=w268) -> ("Maximum"=w267:dynamicdata)  [unwired: 8 in, 2 out]
                n216 = call-poly <vilib>:"Get Waveform Time Array.vi"("waveform in"=w311) -> ("X array"=w316:timestamp[])  [unwired: 9 in, 1 out]
                n217 = call "Derivative (dX/dt)"("Signals"=w272) -> ("Result"=w293:dynamicdata)  [unwired: 5 in, 1 out]
                n218 = call "Convert from Dynamic Data3"("Dynamic Data Type"=w293) -> ("Array"=w292:dbl[])  [unwired: 3 in]
                n219 = To Double Precision Float(number=w316) -> (double precision float=→"double precision float":dbl[])
                n220 = Add(1:w265, 2:w267) -> (0:w270:dynamicdata)  [unwired: 1 in, 1 out]
                n221 = local read "Phase unit"() -> (w310:u16)
                n222 = call "Convert from Dynamic Data15"("Dynamic Data Type"=w270) -> ("Scalar"=w284:dbl)  [unwired: 3 in]
                n223 = call "Convert from Dynamic Data16"("Dynamic Data Type"=w280) -> ("Array"=w279:dbl[])  [unwired: 3 in]
                n224 = call "?"("Dynamic Data Type"=w270) -> ("Array"=w289:dbl[])  [unwired: 3 in]
                n225 = call "Sample Compression50"("Signals"=w293) -> ("Maximum"=w295:dynamicdata)  [unwired: 8 in, 2 out]
                "ROCOF" <- w295
                n226 = Greater?(x=w284, y=0.0) -> (0:w283:bool)
                n227 = case shown="0, Default" w310 {
                  tunnel: w289 -> [w345 w349]
                  tunnel: [w344 w349] -> w281
                  frame 0, Default {
                    n228 = Divide(x=w345, y=3.141592653589793) -> (x/y=w348:dbl[])
                    n229 = Multiply(x=w348, y=180.0) -> (x*y=w344:dbl[])
                  }
                  frame 1 {
                  }
                }
                n230 = call "Convert to Dynamic Data"("Array"=w281) -> ("Dynamic Data Type"=w288:dynamicdata)  [unwired: 3 in]
                n231 = call "Convert from Dynamic Data13"("Dynamic Data Type"=w288) -> ("Array"=w305:dbl[])  [unwired: 3 in]
                n232 = local read "Phase unit"() -> (w282:u16)
                n233 = call "Convert from Dynamic Data10"("Dynamic Data Type"=w295) -> ("Scalar"=w299:dbl)  [unwired: 3 in]
                n234 = case shown="True" w283 {
                  tunnel: w282 -> [w328 w337]
                  tunnel: w281 -> [w327 w336]
                  tunnel: w279 -> [w325 w335]
                  tunnel: [w323 w334] -> w274
                  frame False {
                    n235 = case shown="1" w328 {
                      frame 0, Default {
                        n236 = property on="Phase waveform" class="WFChart (strict)"("YScale.Maximum"=0.0 ("Y Scale.Range:Maximum")) -> ()  [unwired: 2 in, 2 out]
                        n237 = property on="Phase waveform" class="WFChart (strict)"("YScale.Minimum"=-360.0 ("Y Scale.Range:Maximum")) -> ()  [unwired: 2 in, 2 out]
                      }
                      frame 1 {
                        n238 = property on="Phase waveform" class="WFChart (strict)"("YScale.Maximum"=0.0 ("Y Scale.Range:Minimum")) -> ()  [unwired: 2 in, 2 out]
                        n239 = Negate(x=6.283185307179586) -> (-x=w331:dbl)
                        n240 = property on="Phase waveform" class="WFChart (strict)"("YScale.Minimum"=w331) -> ()  [unwired: 2 in, 2 out]
                      }
                    }
                    n241 = Negate(x=w327) -> (-x=w324:dbl[])
                    n242 = Quotient & Remainder(x=w324, y=w325) -> (x-y*floor(x/y)=w326:dbl[])  [unwired: 1 out]
                    n243 = Negate(x=w326) -> (-x=w323:dbl[])
                  }
                  frame True {
                    n244 = case shown="0, Default" w337 {
                      frame 0, Default {
                        n245 = property on="Phase waveform" class="WFChart (strict)"("YScale.Maximum"=360.0 ("Y Scale.Range:Maximum")) -> ()  [unwired: 2 in, 2 out]
                        n246 = property on="Phase waveform" class="WFChart (strict)"("YScale.Minimum"=0.0 ("Y Scale.Range:Maximum")) -> ()  [unwired: 2 in, 2 out]
                      }
                      frame 1 {
                        n247 = property on="Phase waveform" class="WFChart (strict)"("YScale.Maximum"=6.283185307179586) -> ()  [unwired: 2 in, 2 out]
                        n248 = property on="Phase waveform" class="WFChart (strict)"("YScale.Minimum"=0.0 ("Y Scale.Range:Maximum")) -> ()  [unwired: 2 in, 2 out]
                      }
                    }
                    n249 = Quotient & Remainder(x=w336, y=w335) -> (x-y*floor(x/y)=w334:dbl[])  [unwired: 1 out]
                  }
                }
                n250 = In Range and Coerce(upper limit=5.0, x=w299, lower limit=-5.0) -> (coerced(x)=w296:dbl)  [unwired: 1 out]
                n251 = local write "ROCOF waveform 2"(w296) -> ()
                n252 = Unbundle By Name(w264) -> ("t0"=w276:timestamp, "dt"=w278:dbl)
                n253 = Multiply(x=w278, y=2.0) -> (x*y=w275:dbl)
                n254 = Bundle By Name("Y"=w274, "t0"=w276, "dt"=w275) -> (w273:waveform(dbl))  [unwired: 1 in]
                "Phase waveform" <- w273
                n255 = call "Elapsed Time3"() -> ("Time has Elapsed"=w309:bool)  [unwired: 12 in, 7 out]
                n256 = local write "Phase"(w273) -> ()
                n257 = Stop(stop? (T)=w309) -> ()
              }
              frame 1 {
                w357 = FALSE
                w382 = TRUE ("Visible")
                # "voltage step"
                n258 = local read "Sampling info"() -> (w369:cluster{"Fs":dbl, "#s":dbl})
                n259 = call <vilib>:"Formula Waveform.vi"("sampling info"=w369, "formula"="a", "amplitude"=w366) -> ("signal out"=w354:waveform(dbl))  [unwired: 7 in, 1 out]
                n260 = call <vilib>:"Formula Waveform.vi"("sampling info"=w369, "formula"="a", "amplitude"=w367) -> ("signal out"=w359:waveform(dbl))  [unwired: 7 in, 1 out]
                n261 = call "Sample Compression10"("Signals"=w354) -> ("Maximum"=w351:dynamicdata)  [unwired: 8 in, 2 out]
                n262 = call "Elapsed Time"() -> ("Elapsed Time (s)"=w381:dbl)  [unwired: 12 in, 7 out]
                n263 = call "Sample Compression12"("Signals"=w359) -> ("Maximum"=w358:dynamicdata)  [unwired: 8 in, 2 out]
                n264 = call <vilib>:"Formula Waveform.vi"("sampling info"=w369, "formula"="a", "amplitude"=w362) -> ("signal out"=w353:waveform(dbl))  [unwired: 7 in, 1 out]
                n265 = local write "Array 2"(w354) -> ()
                n266 = local write "Phase"(w351) -> ()
                n267 = call "Sample Compression9"("Signals"=w353) -> ("Maximum"=w363:dynamicdata)  [unwired: 8 in, 2 out]
                n268 = call <vilib>:"Formula Waveform.vi"("sampling info"=w369, "formula"="a", "amplitude"=w372) -> ("signal out"=w356:waveform(dbl))  [unwired: 7 in, 1 out]
                n269 = local write "Array 3"(w353) -> ()
                n270 = local write "Frequency waveform"(w363) -> ()
                n271 = call "Sample Compression11"("Signals"=w356) -> ("Maximum"=w364:dynamicdata)  [unwired: 8 in, 2 out]
                n272 = local write "Frequency"(w363) -> ()
                n273 = Less Or Equal?(x=w381, y=0.3) -> (x <= y?=w379:bool)
                n274 = local read "Phase unit"() -> (w352:u16)
                n275 = call <vilib>:"Formula Waveform.vi"("sampling info"=w369, "formula"="a+a*f", "amplitude"=w367, "frequency"="Voltage step") -> ("signal out"=w361:waveform(dbl))  [unwired: 6 in, 1 out]
                n276 = local write "ROCOF"(w364) -> ()
                n277 = case shown="1" w352 {
                  tunnel: w351 -> [w387 w388]
                  tunnel: [w383 w388] -> w350
                  frame 0, Default {
                    n278 = Multiply(x=w387, y=180.0) -> (x*y=w384:dynamicdata)
                    n279 = Divide(x=w384, y=3.141592653589793) -> (x/y=w383:dynamicdata)
                  }
                  frame 1 {
                  }
                }
                n280 = local write "ROCOF waveform"(w364) -> ()
                n281 = call "Sample Compression4"("Signals"=w361) -> ("Maximum"=w360:dynamicdata)  [unwired: 8 in, 2 out]
                n282 = case shown="False" w379 {
                  tunnel: [w390 w392] -> w365
                  tunnel: w358 -> [_ w392]
                  tunnel: w360 -> [w390 _]
                  tunnel: [w389 w391] -> w355
                  tunnel: w359 -> [_ w391]
                  tunnel: w361 -> [w389 _]
                  frame False {
                  }
                  frame True {
                  }
                }
                "Voltage" <- w365
                "Array" <- w355
                n283 = local write "Phase waveform"(w350) -> ()
                n284 = call-poly <vilib>:"Get Waveform Time Array.vi"("waveform in"=w355) -> ("X array"=w376:timestamp[])  [unwired: 9 in, 1 out]
                n285 = local write "Votlage waveform"(w365) -> ()
                n286 = To Double Precision Float(number=w376) -> (double precision float=w377:dbl[])
                n287 = local write "double precision float"(w377) -> ()
                n288 = call "Elapsed Time2"() -> ("Time has Elapsed"=w378:bool)  [unwired: 12 in, 7 out]
                n289 = Stop(stop? (T)=w378) -> ()
              }
              frame 2 {
                w421 = TRUE
                w444 = FALSE ("Visible")
                n290 = local read "Sampling info"() -> (w408:cluster{"Fs":dbl, "#s":dbl})
                n291 = call <vilib>:"Formula Waveform.vi"("sampling info"=w408, "formula"="a", "amplitude"=w432) -> ("signal out"=w415:waveform(dbl))  [unwired: 7 in, 1 out]
                n292 = call-poly <vilib>:"Get Waveform Time Array.vi"("waveform in"=w415) -> ("X array"=w440:timestamp[])  [unwired: 9 in, 1 out]
                n293 = call <vilib>:"Formula Waveform.vi"("sampling info"=w408, "formula"="a", "amplitude"=w430) -> ("signal out"=w420:waveform(dbl))  [unwired: 7 in, 1 out]
                n294 = local write "Array"(w415) -> ()
                n295 = call "Sample Compression14"("Signals"=w415) -> ("Maximum"=w425:dynamicdata)  [unwired: 8 in, 2 out]
                n296 = To Double Precision Float(number=w440) -> (double precision float=w439:dbl[])
                n297 = call "Sample Compression41"("Signals"=w420) -> ("Maximum"=w428:dynamicdata)  [unwired: 8 in, 2 out]
                n298 = local write "Voltage"(w425) -> ()
                n299 = local write "Votlage waveform"(w425) -> ()
                n300 = local write "double precision float"(w439) -> ()
                n301 = call "Elapsed Time4"() -> ("Elapsed Time (s)"=w445:dbl)  [unwired: 12 in, 7 out]
                n302 = call <vilib>:"Formula Waveform.vi"("sampling info"=w408, "formula"="a+1*f", "amplitude"=w430, "frequency"="Phase step") -> ("signal out"=w427:waveform(dbl))  [unwired: 6 in, 1 out]
                n303 = call <vilib>:"Formula Waveform.vi"("sampling info"=w408, "formula"="a", "amplitude"=w414) -> ("signal out"=w395:waveform(dbl))  [unwired: 7 in, 1 out]
                n304 = call <vilib>:"Formula Waveform.vi"("sampling info"=w408, "formula"="a", "amplitude"=w410) -> ("signal out"=w406:waveform(dbl))  [unwired: 7 in, 1 out]
                n305 = Less Or Equal?(x=w445, y=0.3) -> (x <= y?=w409:bool)
                n306 = call "Sample Compression15"("Signals"=w427) -> ("Maximum"=w426:dynamicdata)  [unwired: 8 in, 2 out]
                n307 = call "Sample Compression17"("Signals"=w395) -> ("Maximum"=w412:dynamicdata)  [unwired: 8 in, 2 out]
                n308 = call "Sample Compression18"("Signals"=w406) -> ("Maximum"=w407:dynamicdata)  [unwired: 8 in, 2 out]
                n309 = case shown="False" w409 {
                  tunnel: [w457 w459] -> w398
                  tunnel: w428 -> [_ w459]
                  tunnel: w426 -> [w457 _]
                  tunnel: w420 -> [_ w458]
                  tunnel: [w456 w458] -> w417
                  tunnel: w427 -> [w456 _]
                  frame False {
                  }
                  frame True {
                  }
                }
                "Array 2" <- w417
                n310 = local read "Phase unit"() -> (w397:u16)
                n311 = case shown="0, Default" w397 {
                  tunnel: w398 -> [w446 w447]
                  tunnel: [w446 w447] -> w393
                  frame 0, Default {
                  }
                  frame 1 {
                  }
                }
                "Phase" <- w393
                n312 = Subtract(1:w420, 2:w417) -> (0:w419:waveform(dbl))  [unwired: 1 in, 1 out]
                n313 = call "Derivative (dX/dt)"("Signals"=w419) -> ("Result"=w396:dynamicdata)  [unwired: 5 in, 1 out]
                n314 = Add(1:w395, 2:w396) -> (0:w394:dynamicdata)  [unwired: 1 in, 1 out]
                n315 = local write "Phase waveform"(w393) -> ()
                n316 = call "Sample Compression13"("Signals"=w394) -> ("Maximum"=w400:dynamicdata)  [unwired: 6 in, 4 out]
                n317 = case shown="True" w409 {
                  tunnel: w395 -> [_ w455]
                  tunnel: w412 -> [_ w454]
                  tunnel: [w453 w455] -> w402
                  tunnel: [w452 w454] -> w401
                  tunnel: w394 -> [w453 _]
                  tunnel: w400 -> [w452 _]
                  frame False {
                  }
                  frame True {
                  }
                }
                n318 = call "Convert from Dynamic Data7"("Dynamic Data Type"=w402) -> ("Array"=w416:dbl[])  [unwired: 3 in]
                n319 = call "Derivative (dX/dt)"("Signals"=w402) -> ("Result"=w404:dynamicdata)  [unwired: 5 in, 1 out]
                n320 = call "Elapsed Time5"() -> ("Time has Elapsed"=w443:bool)  [unwired: 12 in, 7 out]
                n321 = call "Convert from Dynamic Data"("Dynamic Data Type"=w401) -> ("Scalar"=w438:dbl)  [unwired: 3 in]
                n322 = call "Sample Compression16"("Signals"=w404) -> ("Maximum"=w399:dynamicdata)  [unwired: 5 in, 5 out]
                n323 = case shown="False" w409 {
                  tunnel: w407 -> [_ w451]
                  tunnel: w406 -> [_ w450]
                  tunnel: [w449 w451] -> w405
                  tunnel: [w448 w450] -> w403
                  tunnel: w399 -> [w449 _]
                  tunnel: w404 -> [w448 _]
                  frame False {
                  }
                  frame True {
                  }
                }
                n324 = call "Convert from Dynamic Data8"("Dynamic Data Type"=w403) -> ("Array"=w418:dbl[])  [unwired: 3 in]
                n325 = call "Convert from Dynamic Data2"("Dynamic Data Type"=w405) -> ("Scalar"=w435:dbl)  [unwired: 3 in]
                n326 = In Range and Coerce(upper limit=5.0, x=w435, lower limit=-5.0) -> (coerced(x)=w422:dbl)  [unwired: 1 out]
                "ROCOF waveform 2" <- w422
                n327 = In Range and Coerce(upper limit=55.0, x=w438, lower limit=45.0) -> (coerced(x)=w423:dbl)  [unwired: 1 out]
                "Frequency waveform 2" <- w423
                n328 = Stop(stop? (T)=w443) -> ()
                n329 = local write "Frequency"(w423) -> ()
                n330 = local write "ROCOF"(w422) -> ()
              }
              frame 3 {
                w498 = TRUE
                w501 = FALSE ("Visible")
                n331 = call "Elapsed Time7"() -> ("Time has Elapsed"=w517:bool)  [unwired: 12 in, 7 out]
                n332 = local read "Sampling info"() -> (w469:cluster{"Fs":dbl, "#s":dbl})
                n333 = call <vilib>:"Formula Waveform.vi"("sampling info"=w469, "formula"="a", "amplitude"=w499) -> ("signal out"=w496:waveform(dbl))  [unwired: 7 in, 1 out]
                n334 = local write "Array"(w496) -> ()
                n335 = call "Sample Compression22"("Signals"=w496) -> ("Maximum"=w502:dynamicdata)  [unwired: 8 in, 2 out]
                n336 = call <vilib>:"Formula Waveform.vi"("sampling info"=w469, "formula"="a", "amplitude"=w508) -> ("signal out"=w506:waveform(dbl))  [unwired: 7 in, 1 out]
                n337 = call <vilib>:"Formula Waveform.vi"("sampling info"=w469, "formula"="a", "amplitude"=w492) -> ("signal out"=w504:waveform(dbl))  [unwired: 7 in, 1 out]
                n338 = Stop(stop? (T)=w517) -> ()
                n339 = call <vilib>:"Formula Waveform.vi"("sampling info"=w469, "formula"="a", "amplitude"=w513) -> ("signal out"=w494:waveform(dbl))  [unwired: 7 in, 1 out]
                n340 = local write "Voltage"(w502) -> ()
                n341 = local write "Votlage waveform"(w502) -> ()
                n342 = call "Sample Compression29"("Signals"=w504) -> ()  [unwired: 8 in, 3 out]
                n343 = call "Sample Compression26"("Signals"=w506) -> ("Maximum"=w505:dynamicdata)  [unwired: 8 in, 2 out]
                n344 = call "Sample Compression20"("Signals"=w494) -> ("Maximum"=w507:dynamicdata)  [unwired: 8 in, 2 out]
                n345 = call <vilib>:"Formula Waveform.vi"("sampling info"=w469, "formula"="a+1*f", "amplitude"=w513, "frequency"="Frequency step") -> ("signal out"=w493:waveform(dbl))  [unwired: 6 in, 1 out]
                n346 = call "Elapsed Time6"() -> ("Elapsed Time (s)"=w520:dbl)  [unwired: 12 in, 7 out]
                n347 = call "Sample Compression27"("Signals"=w493) -> ("Maximum"=w503:dynamicdata)  [unwired: 8 in, 2 out]
                n348 = Less Or Equal?(x=w520, y=0.3) -> (x <= y?=w481:bool)
                n349 = local read "Phase unit"() -> (w471:u16)
                n350 = case shown="0, Default" w471 {
                  tunnel: [361.0 ("amplitude") 6.283185307179586] -> w472
                  frame 0, Default {
                  }
                  frame 1 {
                  }
                }
                n351 = case shown="False" w481 {
                  tunnel: [w567 w569] -> w489
                  tunnel: w507 -> [_ w569]
                  tunnel: w503 -> [w567 _]
                  tunnel: [w566 w568] -> w488
                  tunnel: w494 -> [_ w568]
                  tunnel: w493 -> [w566 _]
                  frame False {
                  }
                  frame True {
                  }
                }
                "Frequency" <- w489
                "Array 3" <- w488
                n352 = Subtract(1:w494, 2:w488) -> (0:w486:waveform(dbl))  [unwired: 1 in, 1 out]
                n353 = call "Derivative (dX/dt)"("Signals"=w486) -> ("Result"=w485:dynamicdata)  [unwired: 5 in, 1 out]
                n354 = call "Sample Compression30"("Signals"=w485) -> ("Mean"=w484:dynamicdata)  [unwired: 8 in, 2 out]
                n355 = call "Convert from Dynamic Data5"("Dynamic Data Type"=w484) -> ("Scalar"=w519:dbl)  [unwired: 3 in]
                n356 = In Range and Coerce(upper limit=5.0, x=w519, lower limit=-5.0) -> (coerced(x)=w500:dbl)  [unwired: 1 out]
                n357 = call "Convert from Dynamic Data4"("Dynamic Data Type"=w485) -> ("Array"=w495:dbl[])  [unwired: 3 in]
                n358 = local write "ROCOF"(w500) -> ()
                n359 = local write "ROCOF waveform 2"(w500) -> ()
                n360 = call <vilib>:"Formula Waveform.vi"("sampling info"=w469, "formula"="a", "amplitude"=360.0) -> ("signal out"=w460:waveform(dbl))  [unwired: 7 in, 1 out]
                n361 = local write "Frequency waveform"(w489) -> ()
                n362 = call-poly <vilib>:"Get Waveform Time Array.vi"("waveform in"=w488) -> ("X array"=w510:timestamp[])  [unwired: 9 in, 1 out]
                n363 = local read "Phase unit"() -> (w476:u16)
                n364 = call "Sample Compression47"("Signals"=w460) -> ("Maximum"=w462:dynamicdata)  [unwired: 8 in, 2 out]
                n365 = To Double Precision Float(number=w510) -> (double precision float=w509:dbl[])
                n366 = Greater?(x="Frequency step", y=0.0) -> (0:w463:bool)
                n367 = case shown="False" w463 {
                  tunnel: w472 -> [w543 w545]
                  tunnel: [w544 w545] -> w468
                  frame False {
                    n368 = Negate(x=w543) -> (-x=w544:dbl)
                  }
                  frame True {
                  }
                }
                n369 = case shown="False" w463 {
                  tunnel: w462 -> [w523 w524]
                  tunnel: [w522 w524] -> w461
                  frame False {
                    n370 = Negate(x=w523) -> (-x=w522:dynamicdata)
                  }
                  frame True {
                  }
                }
                n371 = call "Integral (Sum[Xdt])"("Signals"=w486) -> ("Result"=w478:dynamicdata)  [unwired: 5 in, 1 out]
                n372 = call "Convert from Dynamic Data11"() -> ("Scalar"=w518:dbl)  [unwired: 4 in]
                n373 = case shown="1, Default" w476 {
                  tunnel: [360.0 6.283185307179586] -> w480
                  tunnel: [w553 w555] -> w479
                  frame 0 {
                    n374 = Negate(x=360.0) -> (-x=w553:dbl)
                  }
                  frame 1, Default {
                    n375 = Negate(x=6.283185307179586) -> (-x=w555:dbl)
                  }
                }
                n376 = local write "double precision float"(w509) -> ()
                n377 = In Range and Coerce(upper limit=w480, x=w518, lower limit=w479) -> (coerced(x)=→"Phase waveform 2":dbl)  [unwired: 1 out]
                n378 = case shown="1" w476 {
                  tunnel: w478 -> [w547 w550]
                  tunnel: [w546 w549] -> w477
                  frame 0, Default {
                    n379 = Multiply(x=w547, y=360.0) -> (x*y=w546:dynamicdata)
                  }
                  frame 1 {
                    n380 = Multiply(x=w550, y=6.283185307179586) -> (x*y=w549:dynamicdata)
                  }
                }
                n381 = call "Sample Compression19"("Signals"=w477) -> ("Maximum"=w483:dynamicdata)  [unwired: 8 in, 2 out]
                n382 = case shown="False" w481 {
                  tunnel: [w562 w565] -> w466
                  tunnel: w505 -> [_ w565]
                  tunnel: w477 -> [w563 _]
                  tunnel: w506 -> [_ w564]
                  tunnel: [w563 w564] -> w482
                  tunnel: w483 -> [w562 _]
                  frame False {
                  }
                  frame True {
                  }
                }
                n383 = call "Convert from Dynamic Data6"("Dynamic Data Type"=w482) -> ("Array"=w487:dbl[])  [unwired: 3 in]
                n384 = case shown="False" w481 {
                  tunnel: [w559 w561] -> _
                  tunnel: w505 -> [w559 w560]
                  tunnel: [w558 w560] -> w497
                  tunnel: w506 -> [w558 _]
                  tunnel: w466 -> [_ w561]
                  frame False {
                  }
                  frame True {
                  }
                }
                n385 = for {
                  N: 50 -> [_]
                  tunnel: w468 -> [w529]
                  shift-right: [w526] -> w464
                  shift-left: w466 -> [w527]
                  tunnel: w461 -> [w528]
                  tunnel: w463 -> [w525]
                  n386 = case shown="True" w525 {
                    tunnel: w527 -> [w533 w536]
                    tunnel: [w532 w535] -> w530
                    tunnel: w529 -> [w531 w534]
                    frame False {
                      n387 = Less Or Equal?(x=w533, y=w531) -> (x <= y?=w532:dynamicdata)
                    }
                    frame True {
                      n388 = Greater Or Equal?(x=w536, y=w534) -> (x >= y?=w535:dynamicdata)
                    }
                  }
                  n389 = case shown="True" w530 {
                    tunnel: w527 -> [w537 w540]
                    tunnel: [w537 w538] -> w526
                    tunnel: w528 -> [_ w539]
                    frame False {
                    }
                    frame True {
                      n390 = Subtract(1:w539, 2:w540) -> (0:w538:dynamicdata)  [unwired: 1 in, 1 out]
                    }
                  }
                }
                n391 = local write "Array 2"(w497) -> ()
                n392 = local write "Phase waveform"(w464) -> ()
                n393 = local write "Phase"(w464) -> ()
              }
              frame 4 {
                w631 = TRUE ("Visible")
                w598 = FALSE ("Visible")
                n394 = local read "Phase unit"() -> (w583:u16)
                n395 = local read "Sampling info"() -> (w600:cluster{"Fs":dbl, "#s":dbl})
                n396 = case shown="0, Default" w583 {
                  tunnel: [365.0 ("amplitude") 6.283185307179586] -> w582
                  frame 0, Default {
                  }
                  frame 1 {
                  }
                }
                n397 = call <vilib>:"Formula Waveform.vi"("sampling info"=w600, "formula"="a", "amplitude"="ROCOF rate") -> ("signal out"=w618:waveform(dbl))  [unwired: 7 in, 1 out]
                n398 = local read "Sampling info"() -> (w599:cluster{"Fs":dbl, "#s":dbl})
                n399 = call "Sample Compression36"("Signals"=w618) -> ()  [unwired: 8 in, 3 out]
                n400 = call <vilib>:"Formula Waveform.vi"("sampling info"=w599, "formula"="a", "amplitude"=w602) -> ("signal out"=w596:waveform(dbl))  [unwired: 7 in, 1 out]
                n401 = call <vilib>:"Formula Waveform.vi"("sampling info"=w600, "formula"="a", "amplitude"=w597) -> ("signal out"=w587:waveform(dbl))  [unwired: 7 in, 1 out]
                n402 = call <vilib>:"Formula Waveform.vi"("sampling info"=w600, "formula"="a", "amplitude"=w615) -> ("signal out"=w612:waveform(dbl))  [unwired: 7 in, 1 out]
                n403 = call <vilib>:"Formula Waveform.vi"("sampling info"=w600, "formula"="a", "amplitude"=360.0) -> ("signal out"=w579:waveform(dbl))  [unwired: 7 in, 1 out]
                n404 = call "Sample Compression32"("Signals"=w596) -> ("Maximum"=w601:dynamicdata)  [unwired: 8 in, 2 out]
                n405 = local write "Array"(w596) -> ()
                n406 = call "Elapsed Time10"() -> ("Elapsed Time (s)"=w629:dbl)  [unwired: 12 in, 7 out]
                n407 = call "Sample Compression37"("Signals"=w612) -> ("Maximum"=w613:dynamicdata)  [unwired: 8 in, 2 out]
                n408 = call "Sample Compression40"("Signals"=w579) -> ("Maximum"=w571:dynamicdata)  [unwired: 8 in, 2 out]
                n409 = call "Sample Compression34"("Signals"=w587) -> ("Maximum"=w620:dynamicdata)  [unwired: 8 in, 2 out]
                n410 = Less Or Equal?(x=w629, y=0.3) -> (x <= y?=w616:bool)
                n411 = Greater?(x="ROCOF rate", y=0.0) -> (0:w610:bool)
                n412 = local write "Votlage waveform"(w601) -> ()
                n413 = local write "Voltage"(w601) -> ()
                n414 = call <vilib>:"Formula Waveform.vi"("sampling info"=w600, "formula"="a", "amplitude"="Final freq.") -> ("signal out"=w588:waveform(dbl))  [unwired: 7 in, 1 out]
                n415 = call "Sample Compression33"("Signals"=w588) -> ("Maximum"=w625:dynamicdata)  [unwired: 8 in, 2 out]
                n416 = Greater?(x="ROCOF rate", y=0.0) -> (0:w572:bool)
                n417 = case shown="False" w572 {
                  tunnel: w582 -> [w657 w659]
                  tunnel: [w658 w659] -> w576
                  frame False {
                    n418 = Negate(x=w657) -> (-x=w658:dbl)
                  }
                  frame True {
                  }
                }
                n419 = call <vilib>:"Formula Waveform.vi"("sampling info"=w600, "formula"="(a-0.3*f)+f*t", "amplitude"=w597, "frequency"="ROCOF rate") -> ("signal out"=w605:waveform(dbl))  [unwired: 6 in, 1 out]
                n420 = call "Sample Compression31"("Signals"=w605) -> ("Maximum"=w604:dynamicdata)  [unwired: 8 in, 2 out]
                n421 = case shown="False" w610 {
                  tunnel: w604 -> [w662 w665]
                  tunnel: "Final freq." -> [w661 w664]
                  tunnel: [w660 w663] -> w608
                  frame False {
                    n422 = Greater?(x=w662, y=w661) -> (0:w660:dynamicdata)
                  }
                  frame True {
                    n423 = Less?(x=w665, y=w664) -> (x < y?=w663:dynamicdata)
                  }
                }
                n424 = case shown="False" w616 {
                  tunnel: w620 -> [_ w673]
                  tunnel: w587 -> [_ w672]
                  tunnel: [w671 w673] -> w623
                  tunnel: [w670 w672] -> w589
                  tunnel: w604 -> [w671 _]
                  tunnel: w605 -> [w670 _]
                  frame False {
                  }
                  frame True {
                  }
                }
                n425 = case shown="True" w608 {
                  tunnel: [w675 w677] -> w595
                  tunnel: w625 -> [w675 _]
                  tunnel: [w674 w676] -> w594
                  tunnel: w588 -> [w674 _]
                  tunnel: w623 -> [_ w677]
                  tunnel: w589 -> [_ w676]
                  frame False {
                  }
                  frame True {
                  }
                }
                n426 = case shown="False" w572 {
                  tunnel: w571 -> [w633 w634]
                  tunnel: [w632 w634] -> w570
                  frame False {
                    n427 = Negate(x=w633) -> (-x=w632:dynamicdata)
                  }
                  frame True {
                  }
                }
                n428 = local read "Phase unit"() -> (w586:u16)
                n429 = Subtract(1:w587, 2:w594) -> (0:w593:waveform(dbl))  [unwired: 1 in, 1 out]
                n430 = call "Integral (Sum[Xdt])"("Signals"=w593) -> ("Result"=w585:dynamicdata)  [unwired: 5 in, 1 out]
                n431 = case shown="0, Default" w586 {
                  tunnel: w585 -> [w655 w656]
                  tunnel: [w653 w656] -> w584
                  frame 0, Default {
                    n432 = Multiply(x=w655, y=360.0) -> (x*y=w653:dynamicdata)
                  }
                  frame 1 {
                  }
                }
                n433 = call-poly <vilib>:"Get Waveform Time Array.vi"("waveform in"=w594) -> ("X array"=w622:timestamp[])  [unwired: 9 in, 1 out]
                n434 = local write "Frequency waveform"(w595) -> ()
                n435 = local write "Array 3"(w594) -> ()
                n436 = local write "Frequency"(w595) -> ()
                n437 = call "Derivative (dX/dt)"("Signals"=w593) -> ("Result"=w581:dynamicdata)  [unwired: 5 in, 1 out]
                n438 = call "Convert from Dynamic Data12"("Dynamic Data Type"=w581) -> ("Array"=w580:dbl[])  [unwired: 3 in]
                n439 = To Double Precision Float(number=w622) -> (double precision float=w621:dbl[])
                n440 = local write "double precision float"(w621) -> ()
                n441 = call "Elapsed Time8"() -> ("Time has Elapsed"=w628:bool)  [unwired: 12 in, 7 out]
                n442 = call "Sample Compression28"("Signals"=w581) -> ("Maximum"=w573:dynamicdata)  [unwired: 8 in, 2 out]
                n443 = call "Sample Compression39"("Signals"=w584) -> ("Maximum"=w592:dynamicdata)  [unwired: 8 in, 2 out]
                n444 = case shown="False" w616 {
                  tunnel: w613 -> [_ w669]
                  tunnel: [w667 w669] -> w577
                  tunnel: w612 -> [_ w668]
                  tunnel: [w666 w668] -> w590
                  tunnel: w592 -> [w667 _]
                  tunnel: w584 -> [w666 _]
                  frame False {
                  }
                  frame True {
                  }
                }
                n445 = call "Convert from Dynamic Data9"("Dynamic Data Type"=w590) -> ("Array"=w591:dbl[])  [unwired: 3 in]
                n446 = for {
                  N: 50 -> [_]
                  tunnel: w576 -> [w639]
                  shift-right: [w636] -> w575
                  shift-left: w577 -> [w637]
                  tunnel: w570 -> [w638]
                  tunnel: w572 -> [w635]
                  n447 = case shown="True" w635 {
                    tunnel: w637 -> [w643 w646]
                    tunnel: [w642 w645] -> w640
                    tunnel: w639 -> [w641 w644]
                    frame False {
                      n448 = Less Or Equal?(x=w643, y=w641) -> (x <= y?=w642:dynamicdata)
                    }
                    frame True {
                      n449 = Greater?(x=w646, y=w644) -> (0:w645:dynamicdata)
                    }
                  }
                  n450 = case shown="True" w640 {
                    tunnel: w637 -> [w647 w650]
                    tunnel: [w647 w648] -> w636
                    tunnel: w638 -> [_ w649]
                    frame False {
                    }
                    frame True {
                      n451 = Subtract(1:w649, 2:w650) -> (0:w648:dynamicdata)  [unwired: 1 in, 1 out]
                    }
                  }
                }
                n452 = Stop(stop? (T)=w628) -> ()
                n453 = local write "ROCOF waveform"(w573) -> ()
                n454 = local write "ROCOF"(w573) -> ()
                n455 = local write "Phase waveform"(w575) -> ()
                n456 = local write "Phase"(w575) -> ()
              }
              frame 5 {
                w711 = TRUE
                w686 = FALSE
                n457 = call "Elapsed Time11"() -> ("Elapsed Time (s)"=w710:dbl)  [unwired: 12 in, 7 out]
                n458 = Less Or Equal?(x=w710, y=0.3) -> (x <= y?=w708:bool)
                n459 = call <vilib>:"Formula Waveform.vi"("sampling info"="Sampling info", "formula"="a", "amplitude"=w700) -> ("signal out"=w684:waveform(dbl))  [unwired: 7 in, 1 out]
                n460 = call <vilib>:"Formula Waveform.vi"("sampling info"="Sampling info", "formula"="a", "amplitude"=w703) -> ("signal out"=w682:waveform(dbl))  [unwired: 7 in, 1 out]
                n461 = call <vilib>:"Formula Waveform.vi"("sampling info"="Sampling info", "formula"="a", "amplitude"=w699) -> ("signal out"=w683:waveform(dbl))  [unwired: 7 in, 1 out]
                n462 = local write "Array 2"(w682) -> ()
                n463 = call "Sample Compression"("Signals"=w682) -> ("Maximum"=w679:dynamicdata)  [unwired: 8 in, 2 out]
                n464 = local write "Array 3"(w684) -> ()
                n465 = call "Sample Compression23"("Signals"=w684) -> ("Maximum"=w685:dynamicdata)  [unwired: 8 in, 2 out]
                n466 = call "Sample Compression24"("Signals"=w683) -> ("Maximum"=w698:dynamicdata)  [unwired: 8 in, 2 out]
                n467 = call <vilib>:"Formula Waveform.vi"("sampling info"="Sampling info", "formula"="a", "amplitude"=w688) -> ("signal out"=w692:waveform(dbl))  [unwired: 7 in, 1 out]
                n468 = local read "Phase unit"() -> (w680:u16)
                n469 = call <vilib>:"Formula Waveform.vi"("offset"=w688, "sampling info"="Sampling info", "formula"="a*sin(2*pi(1)*f*t)", "amplitude"="Mod Amp", "frequency"="Mod Freq") -> ("signal out"=w693:waveform(dbl))  [unwired: 5 in, 1 out]
                n470 = local write "Frequency waveform"(w685) -> ()
                n471 = local write "ROCOF waveform"(w698) -> ()
                n472 = call "Sample Compression21"("Signals"=w693) -> ("Maximum"=w690:dynamicdata)  [unwired: 8 in, 2 out]
                n473 = call "Sample Compression43"("Signals"=w692) -> ("Maximum"=w691:dynamicdata)  [unwired: 8 in, 2 out]
                n474 = case shown="True" w708 {
                  tunnel: w688 -> [_ _]
                  tunnel: [w719 w721] -> w681
                  tunnel: w692 -> [_ w721]
                  tunnel: w693 -> [w719 _]
                  tunnel: w691 -> [_ w720]
                  tunnel: [w718 w720] -> w689
                  tunnel: w690 -> [w718 _]
                  frame False {
                  }
                  frame True {
                  }
                }
                n475 = case shown="1" w680 {
                  tunnel: w679 -> [w716 w717]
                  tunnel: [w712 w717] -> w678
                  frame 0, Default {
                    n476 = Multiply(x=w716, y=180.0) -> (x*y=w713:dynamicdata)
                    n477 = Divide(x=w713, y=3.141592653589793) -> (x/y=w712:dynamicdata)
                  }
                  frame 1 {
                  }
                }
                n478 = local write "Phase"(w679) -> ()
                n479 = local write "Frequency"(w685) -> ()
                n480 = local write "ROCOF"(w698) -> ()
                n481 = local write "Phase waveform"(w678) -> ()
                n482 = local write "Votlage waveform"(w689) -> ()
                n483 = local write "Array"(w681) -> ()
                n484 = call-poly <vilib>:"Get Waveform Time Array.vi"("waveform in"=w682) -> ("X array"=w706:timestamp[])  [unwired: 9 in, 1 out]
                n485 = local write "Voltage"(w681) -> ()
                n486 = To Double Precision Float(number=w706) -> (double precision float=w705:dbl[])
                n487 = local write "double precision float"(w705) -> ()
                n488 = call "Elapsed Time9"() -> ("Time has Elapsed"=w707:bool)  [unwired: 12 in, 7 out]
                n489 = Stop(stop? (T)=w707) -> ()
              }
              frame 6 {
                w765 = TRUE
                w732 = FALSE
                n490 = call "Elapsed Time12"() -> ("Elapsed Time (s)"=w763:dbl)  [unwired: 12 in, 7 out]
                n491 = local read "Sampling info"() -> (w736:cluster{"Fs":dbl, "#s":dbl})
                n492 = Less Or Equal?(x=w763, y=0.3) -> (x <= y?=w753:bool)
                n493 = call <vilib>:"Formula Waveform.vi"("sampling info"=w736, "formula"="a", "amplitude"=w759) -> ("signal out"=w725:waveform(dbl))  [unwired: 7 in, 1 out]
                n494 = call "Sample Compression25"("Signals"=w725) -> ("Maximum"=w758:dynamicdata)  [unwired: 8 in, 2 out]
                n495 = Multiply(x="Mod Amp", y="Mod Freq") -> (x*y=→"Freq Dev":dbl)
                n496 = call <vilib>:"Formula Waveform.vi"("sampling info"=w736, "formula"="a", "amplitude"=w734) -> ("signal out"=w750:waveform(dbl))  [unwired: 7 in, 1 out]
                n497 = call <vilib>:"Formula Waveform.vi"("offset"=w734, "sampling info"=w736, "formula"="a*cos(2*pi(1)*f*t-pi(1))", "amplitude"="Mod Amp", "frequency"="Mod Freq") -> ("signal out"=w749:waveform(dbl))  [unwired: 5 in, 1 out]
                n498 = call <vilib>:"Formula Waveform.vi"("offset"=w735, "sampling info"=w736, "formula"="-a*f*sin(2*pi(1)*f*t-pi(1))", "amplitude"="Mod Amp", "frequency"="Mod Freq") -> ("signal out"=w745:waveform(dbl))  [unwired: 5 in, 1 out]
                n499 = call <vilib>:"Formula Waveform.vi"("sampling info"=w736, "formula"="a", "amplitude"=w735) -> ("signal out"=w746:waveform(dbl))  [unwired: 7 in, 1 out]
                n500 = call <vilib>:"Formula Waveform.vi"("sampling info"=w736, "formula"="a", "amplitude"=w733) -> ("signal out"=w741:waveform(dbl))  [unwired: 7 in, 1 out]
                n501 = call <vilib>:"Formula Waveform.vi"("offset"=w733, "sampling info"=w736, "formula"="-a*2*pi(1)*f*f*cos(2*pi(1)*f*t-pi(1))", "amplitude"="Mod Amp", "frequency"="Mod Freq") -> ("signal out"=w740:waveform(dbl))  [unwired: 5 in, 1 out]
                n502 = local write "Array"(w725) -> ()
                n503 = local write "Voltage"(w758) -> ()
                n504 = call "Sample Compression2"("Signals"=w750) -> ("Maximum"=w748:dynamicdata)  [unwired: 8 in, 2 out]
                n505 = call "Sample Compression42"("Signals"=w746) -> ("Maximum"=w743:dynamicdata)  [unwired: 8 in, 2 out]
                n506 = call "Sample Compression44"("Signals"=w741) -> ("Maximum"=w738:dynamicdata)  [unwired: 8 in, 2 out]
                n507 = call-poly <vilib>:"Get Waveform Time Array.vi"("waveform in"=w725) -> ("X array"=w762:timestamp[])  [unwired: 9 in, 1 out]
                n508 = local write "Votlage waveform"(w758) -> ()
                n509 = To Double Precision Float(number=w762) -> (double precision float=w761:dbl[])
                n510 = call "Sample Compression45"("Signals"=w749) -> ("Maximum"=w747:dynamicdata)  [unwired: 8 in, 2 out]
                n511 = case shown="True" w753 {
                  tunnel: [w782 w784] -> w728
                  tunnel: w750 -> [_ w784]
                  tunnel: w749 -> [w782 _]
                  tunnel: [w781 w783] -> w723
                  tunnel: w748 -> [_ w783]
                  tunnel: w747 -> [w781 _]
                  frame False {
                  }
                  frame True {
                  }
                }
                n512 = call "Sample Compression46"("Signals"=w745) -> ("Maximum"=w744:dynamicdata)  [unwired: 8 in, 2 out]
                n513 = case shown="True" w753 {
                  tunnel: [w778 w780] -> w726
                  tunnel: w746 -> [_ w780]
                  tunnel: w745 -> [w778 _]
                  tunnel: [w777 w779] -> w742
                  tunnel: w744 -> [w777 _]
                  tunnel: w743 -> [_ w779]
                  frame False {
                  }
                  frame True {
                  }
                }
                n514 = local write "double precision float"(w761) -> ()
                n515 = call "Sample Compression3"("Signals"=w740) -> ("Maximum"=w739:dynamicdata)  [unwired: 8 in, 2 out]
                n516 = case shown="True" w753 {
                  tunnel: [w774 w776] -> w727
                  tunnel: w741 -> [_ w776]
                  tunnel: w740 -> [w774 _]
                  tunnel: [w773 w775] -> w737
                  tunnel: w739 -> [w773 _]
                  tunnel: w738 -> [_ w775]
                  frame False {
                  }
                  frame True {
                  }
                }
                n517 = local read "Phase unit"() -> (w724:u16)
                n518 = case shown="0, Default" w724 {
                  tunnel: w723 -> [w771 w772]
                  tunnel: [w767 w772] -> w722
                  frame 0, Default {
                    n519 = Multiply(x=w771, y=180.0) -> (x*y=w768:dynamicdata)
                    n520 = Divide(x=w768, y=3.141592653589793) -> (x/y=w767:dynamicdata)
                  }
                  frame 1 {
                  }
                }
                n521 = local write "Frequency waveform"(w742) -> ()
                n522 = local write "Array 2"(w728) -> ()
                n523 = local write "Phase"(w728) -> ()
                n524 = local write "ROCOF"(w727) -> ()
                n525 = local write "ROCOF waveform"(w737) -> ()
                n526 = local write "Frequency"(w726) -> ()
                n527 = local write "Array 3"(w726) -> ()
                n528 = local write "Phase waveform"(w722) -> ()
                n529 = call "Elapsed Time13"() -> ("Time has Elapsed"=w764:bool)  [unwired: 12 in, 7 out]
                n530 = Stop(stop? (T)=w764) -> ()
              }
              frame 7 {
                w785 = dbl[] []
                w786 = FALSE
                w788 = TRUE
                n531 = local write "Voltage"(w787) -> ()
                n532 = local write "Frequency"(w789) -> ()
              }
            }
          }
        }
        n533 = case shown="True" w166 {
          tunnel: [w180 w204] -> w172
          tunnel: [w181 w197] -> w171
          tunnel: w174 -> [w181 w188]
          tunnel: w173 -> [w180 w187]
          tunnel: w169 -> [_ w185]
          tunnel: w170 -> [_ w184]
          tunnel: w168 -> [_ w183]
          tunnel: w167 -> [_ w182]
          frame False {
          }
          frame True {
            w189 = "3 Phase Generator" ("group name in (Untitled)")
            n534 = local read "double precision float"() -> (w186:dbl[])
            n535 = Build Array(w184) -> (w200:dbl[][])
            n536 = Build Array(w183) -> (w199:dbl[][])
            n537 = Build Array(w182) -> (w198:dbl[][])
            n538 = Build Array(w185) -> (w208:dbl[][])
            n539 = TDMS Write(0:w188, 5:w189, 7:"Time" ("channel name(s) in (Untitled)"), 9:w186, 11:w187) -> (4:w192:refnum<k34>, 15:w191:errorcluster)  [unwired: 1 in, 2 out]
            n540 = TDMS Write(0:w192, 5:w189, 7:string[] ["Voltage"] ("channel name(s) in (Untitled)"), 9:w208, 11:w191) -> (4:w203:refnum<k34>, 15:w207:errorcluster)  [unwired: 1 in, 2 out]
            n541 = TDMS Write(0:w203, 5:w189, 7:string[] ["Phase"] ("channel name(s) in (Untitled)"), 9:w200, 11:w207) -> (4:w202:refnum<k34>, 15:w206:errorcluster)  [unwired: 1 in, 2 out]
            n542 = TDMS Write(0:w202, 5:w189, 7:string[] ["Frequency"] ("channel name(s) in (Untitled)"), 9:w199, 11:w206) -> (4:w201:refnum<k34>, 15:w205:errorcluster)  [unwired: 1 in, 2 out]
            n543 = TDMS Write(0:w201, 5:w189, 7:string[] ["ROCOF"] ("channel name(s) in (Untitled)"), 9:w198, 11:w205) -> (4:w197:refnum<k34>, 15:w204:errorcluster)  [unwired: 1 in, 2 out]
          }
        }
        n544 = property on="Mod Freq" class="DigNum (strict)"("Visible"=w161) -> ()  [unwired: 2 in, 2 out]
        n545 = property on="Initial freq." class="DigNum (strict)"("Visible"=w159) -> ()  [unwired: 2 in, 2 out]
        n546 = property on="FreqDev" class="Str"("Visible"=w161) -> ()  [unwired: 2 in, 2 out]
        n547 = property on="Final freq." class="DigNum (strict)"("Visible"=w159) -> ()  [unwired: 2 in, 2 out]
        n548 = property on="Phase waveform 2" class="WFChart (strict)"("Visible"=w164) -> ()  [unwired: 2 in, 2 out]
        n549 = property on="H2 order" class="DigNum (strict)"("Visible"=w164) -> ()  [unwired: 2 in, 2 out]
        n550 = property on="Freq Dev" class="DigNum (strict)"("Visible"=w161) -> ()  [unwired: 2 in, 2 out]
        n551 = property on="H2 Volt" class="DigNum (strict)"("Visible"=w164) -> ()  [unwired: 2 in, 2 out]
        n552 = property on="H2 Phase" class="DigNum (strict)"("Visible"=w164) -> ()  [unwired: 2 in, 2 out]
        n553 = property on="H1 order" class="DigNum (strict)"("Visible"=w164) -> ()  [unwired: 2 in, 2 out]
        n554 = property on="H1 Phase" class="DigNum (strict)"("Visible"=w164) -> ()  [unwired: 2 in, 2 out]
        n555 = property on="Mod Freq" class="DigNum (strict)"("Visible"=w162) -> ()  [unwired: 2 in, 2 out]
        n556 = property on="H1 Volt" class="DigNum (strict)"("Visible"=w164) -> ()  [unwired: 2 in, 2 out]
        n557 = property on="ROCOF rate" class="DigNum (strict)"("Visible"=w159) -> ()  [unwired: 2 in, 2 out]
        n558 = property on="ROCOF waveform 2" class="WFChart (strict)"("Visible"=w175) -> ()  [unwired: 2 in, 2 out]
        n559 = property class="Str"("Visible"=w162) -> ()  [unwired: 2 in, 2 out]
        n560 = property on="Phase step" class="DigNum (strict)"("Visible"=w163) -> ()  [unwired: 2 in, 2 out]
        n561 = property on="Frequency" class="DigNum (strict)"("Visible"=w176) -> ()  [unwired: 2 in, 2 out]
        n562 = property on="2" class="WFChart (strict)"("Visible"=w177) -> ()  [unwired: 2 in, 2 out]
        n563 = property on="Mod Amp" class="DigNum (strict)"("Visible"=w161) -> ()  [unwired: 2 in, 2 out]
        n564 = property on="Mod Amp" class="DigNum (strict)"("Visible"=w162) -> ()  [unwired: 2 in, 2 out]
        n565 = property on="PMFeq" class="Str"("Visible"=w161) -> ()  [unwired: 2 in, 2 out]
        n566 = property on="Time" class="DigNum (strict)"("Visible"=w159) -> ()  [unwired: 2 in, 2 out]
        n567 = property on="second" class="Str"("Visible"=w159) -> ()  [unwired: 2 in, 2 out]
        n568 = property on="Final freq" class="Str"("Visible"=w159) -> ()  [unwired: 2 in, 2 out]
        n569 = property on="Hz/s" class="Str"("Visible"=w159) -> ()  [unwired: 2 in, 2 out]
        n570 = property on="Voltage step" class="DigNum (strict)"("Visible"=w158) -> ()  [unwired: 2 in, 2 out]
        n571 = property on="Frequency step" class="DigNum (strict)"("Visible"=w165) -> ()  [unwired: 2 in, 2 out]
        n572 = property class="Str"("Visible"=w165) -> ()  [unwired: 2 in, 2 out]
      }
      frame #3 {
        n573 = case shown="True" w790 {
          frame False {
          }
          frame True {
            w879 = u8 0  # U8
            n574 = local read "Select test type"() -> (w882:u16)
            n575 = case shown="0, Default" w882 {
              tunnel: [0 1 2 3 4 5 6 7] -> w831
              tunnel: [w905 w914 w926 w948 w981 w1002 w1020 w1043] -> w856
              tunnel: [w904 w913 w925 w947 w980 w1001 w1019 w1024] -> w862
              tunnel: [w903 w912 w924 w946 w979 w1000 w1018 w1042] -> w881
              tunnel: [w902 w908 w917 w939 w971 w997 w1015 w1041] -> w830
              tunnel: [w902 w907 w916 w945 w961 w982 w1004 w1035] -> w828
              tunnel: [w902 w907 w916 w945 w965 w995 w1005 w1045] -> w826
              tunnel: [w902 w907 w916 w945 w965 w982 w1004 w1030] -> w824
              frame 0, Default {
                w902 = 0.0
                n576 = local read "Frequency"() -> (w903:dbl)
                n577 = local read "Phase"() -> (w904:dbl)
                n578 = local read "Voltage"() -> (w905:dbl)
              }
              frame 1 {
                w907 = 0.0
                n579 = local read "Voltage"() -> (w909:dbl)
                n580 = local read "Phase"() -> (w913:dbl)
                n581 = local read "Frequency"() -> (w912:dbl)
                n582 = local read "Voltage"() -> (w914:dbl)
                n583 = Multiply(x=w909, y=52428.8) -> (x*y=w911:dbl)
                n584 = Round Toward +Infinity(x=w911) -> (ceil(x): smallest int >= x=w908:dbl)
              }
              frame 2 {
                w916 = 0.0
                n585 = local read "Phase"() -> (w918:dbl)
                n586 = local read "Phase"() -> (w925:dbl)
                n587 = Divide(x=w918, y=360.0) -> (x/y=w920:dbl)
                n588 = local read "Frequency"() -> (w924:dbl)
                n589 = Power Of X(1:2.0 ("x"), 2:16.0 ("y")) -> (0:w919:dbl)
                n590 = local read "Voltage"() -> (w926:dbl)
                n591 = Multiply(x=w919, y=w920) -> (x*y=w917:dbl)
              }
              frame 3 {
                w945 = 0.0
                n592 = local read "Frequency"() -> (w929:dbl)
                n593 = Power Of X(1:2.0 ("x"), 2:31.0 ("y")) -> (0:w934:dbl)
                n594 = local read "Phase"() -> (w947:dbl)
                n595 = local read "Frequency"() -> (w946:dbl)
                n596 = Power Of X(1:10.0 ("x"), 2:6.0 ("y")) -> (0:w936:dbl)
                n597 = local read "Voltage"() -> (w948:dbl)
                n598 = Multiply(x=w929, y=w934) -> (x*y=w937:dbl)
                n599 = Multiply(x=2.5, y=w936) -> (x*y=w938:dbl)
                n600 = Divide(x=w937, y=w938) -> (x/y=w928:dbl)
                n601 = Round Toward +Infinity(x=w928) -> (ceil(x): smallest int >= x=w944:dbl)
                n602 = Number To Hexadecimal String(2:w944) -> (0:w943:string)  [unwired: 1 in]
                n603 = String Subset(string=w943, offset (0)=0, length (rest)=4 ("length (rest)")) -> (substring=w940:string)
                n604 = Hexadecimal String To Number(string=w940) -> (number=w939:u32)  [unwired: 2 in, 1 out]
              }
              frame 4 {
                w965 = 0.0
                n605 = local read "Final freq."() -> (w958:dbl)
                n606 = local read "ROCOF rate"() -> (w956:dbl)
                n607 = local read "Frequency"() -> (w950:dbl)
                n608 = Power Of X(1:10.0 ("x"), 2:6.0 ("y")) -> (0:w969:dbl)
                n609 = Power Of X(1:2.0 ("x"), 2:42.0 ("y")) -> (0:w974:dbl)
                n610 = local read "Frequency"() -> (w979:dbl)
                n611 = local read "Phase"() -> (w980:dbl)
                n612 = Subtract(x=w958, y=w950) -> (x-y=w957:dbl)
                n613 = local read "Voltage"() -> (w981:dbl)
                n614 = Divide(x=2500000.0, y=64.0) -> (x/y=w975:dbl)
                n615 = Multiply(x=w957, y=w956) -> (x*y=w955:dbl)
                "Time" <- w955
                n616 = Multiply(x=w955, y=w969) -> (x*y=w966:dbl)
                n617 = Multiply(x=2.5, y=w966) -> (x*y=w952:dbl)
                n618 = Multiply(x=w956, y=w974) -> (x*y=w973:dbl)
                n619 = Square(x=w975) -> (x^2=w972:dbl)
                n620 = Divide(x=w952, y=1024.0) -> (x/y=w951:dbl)
                n621 = Number To Hexadecimal String(2:w951) -> (0:w963:string)  [unwired: 1 in]
                n622 = Divide(x=w973, y=w972) -> (x/y=w971:dbl)
                n623 = String Subset(string=w963, offset (0)=0, length (rest)=4 ("length (rest)")) -> (substring=w962:string)
                n624 = Hexadecimal String To Number(string=w962) -> (number=w961:u32)  [unwired: 2 in, 1 out]
              }
              frame 5 {
                w982 = 0.0 ("Frequency")
                n625 = local read "Mod Amp"() -> (w999:dbl)
                n626 = local read "Mod Freq"() -> (w987:dbl)
                n627 = local read "Phase"() -> (w1001:dbl)
                n628 = local read "Frequency"() -> (w1000:dbl)
                n629 = local read "Voltage"() -> (w1002:dbl)
                n630 = Multiply(x=w987, y=68719476736.0) -> (x*y=w984:dbl)
                n631 = Divide(x=w984, y=2500000.0) -> (x/y=w983:dbl)
                n632 = Multiply(x=w999, y=41943.04) -> (x*y=w990:dbl)
                n633 = Multiply(x=10.0, y=w990) -> (x*y=w989:dbl)
                n634 = Format Into String(format string="%4x", w983) -> (resulting string=w994:string)  [unwired: 2 in, 1 out]
                n635 = Round Toward -Infinity(1:w989) -> (0:w997:dbl)
                n636 = String Subset(string=w994, offset (0)=0, length (rest)=4 ("length (rest)")) -> (substring=w991:string)
                n637 = Hexadecimal String To Number(string=w991) -> (number=w995:u32)  [unwired: 2 in, 1 out]
              }
              frame 6 {
                w1004 = 0.0
                n638 = local read "Mod Freq"() -> (w1009:dbl)
                n639 = local read "Mod Amp"() -> (w1016:dbl)
                n640 = local read "Phase"() -> (w1019:dbl)
                n641 = local read "Frequency"() -> (w1018:dbl)
                n642 = local read "Voltage"() -> (w1020:dbl)
                n643 = Multiply(x=w1009, y=68719476736.0) -> (x*y=w1006:dbl)
                n644 = Divide(x=w1006, y=2500000.0) -> (x/y=w1005:dbl)
                n645 = Multiply(x=w1016, y=17179869184.0) -> (x*y=w1012:dbl)
                n646 = Multiply(x=50.0, y=w1012) -> (x*y=w1010:dbl)
                n647 = Divide(x=w1010, y=2500000.0) -> (x/y=w1013:dbl)
                n648 = Round Toward +Infinity(x=w1013) -> (ceil(x): smallest int >= x=w1015:dbl)
              }
              frame 7 {
                n649 = local read "H1 Volt"() -> (w1026:dbl)
                n650 = local read "H2 order"() -> (w1033:dbl)
                n651 = local read "H1 order"() -> (w1034:dbl)
                n652 = local read "H2 Volt"() -> (w1038:dbl)
                n653 = Power Of X(1:2.0 ("x"), 2:16.0 ("y")) -> (0:w1023:dbl)
                n654 = local read "Frequency"() -> (w1042:dbl)
                n655 = local read "Voltage"() -> (w1043:dbl)
                n656 = local read "H1 Phase"() -> (w1041:dbl)
                n657 = local read "H2 Phase"() -> (w1045:dbl)
                n658 = Multiply(x=w1026, y=52428.8) -> (x*y=w1039:dbl)
                n659 = Multiply(x=w1038, y=52428.8) -> (x*y=w1036:dbl)
                n660 = Round Toward +Infinity(x=w1039) -> (ceil(x): smallest int >= x=w1025:dbl)
                n661 = Multiply(x=w1025, y=360.0) -> (x*y=w1022:dbl)
                n662 = Divide(x=w1022, y=w1023) -> (x/y=w1024:dbl)
                n663 = Round Toward +Infinity(x=w1036) -> (ceil(x): smallest int >= x=w1035:dbl)
                n664 = Format Into String(format string="%02x%02x", w1034, w1033) -> (resulting string=w1031:string)  [unwired: 2 in, 1 out]
                n665 = Hexadecimal String To Number(string=w1031) -> (number=w1030:u32)  [unwired: 2 in, 1 out]
              }
            }
            n666 = local read "Phase"() -> (w792:dbl)
            n667 = local read "Voltage"() -> (w798:dbl)
            n668 = local read "Phase unit"() -> (w793:u16)
            n669 = case shown="1" w793 {
              tunnel: w792 -> [w890 w895]
              tunnel: [w890 w891] -> w791
              frame 0, Default {
              }
              frame 1 {
                n670 = Divide(x=w895, y=6.283185307179586) -> (x/y=w893:dbl)
                n671 = Multiply(x=w893, y=360.0) -> (x*y=w891:dbl)
              }
            }
            n672 = Multiply(x=w856, y=52428.8) -> (x*y=w855:dbl)
            n673 = Power Of X(1:2.0 ("x"), 2:16.0 ("y")) -> (0:w859:dbl)
            n674 = call "Convert dec to hex.vi"("P.u. Voltage"=w881) -> ("Numeric"=w853:dbl)  [unwired: 10 in]
            n675 = Divide(x=w862, y=360.0) -> (x/y=w860:dbl)
            n676 = Round Toward +Infinity(x=w855) -> (ceil(x): smallest int >= x=w794:dbl)
            n677 = Multiply(x=w859, y=w860) -> (x*y=w854:dbl)
            n678 = To Long Integer(number=w854) -> (32bit integer=w849:i32)
            n679 = To Long Integer(number=w853) -> (32bit integer=w851:i32)
            n680 = To Long Integer(number=w794) -> (32bit integer=w850:i32)
            n681 = To Long Integer(number=w830) -> (32bit integer=w829:i32)
            n682 = To Long Integer(number=w828) -> (32bit integer=w827:i32)
            n683 = To Long Integer(number=w826) -> (32bit integer=w825:i32)
            n684 = To Long Integer(number=w824) -> (32bit integer=w823:i32)
            n685 = Format Into String(format string="%1x%1x%6x%4x%4x%4x%04x%04x%04x", "Data type", w831, w851, w850, w849, w829, w827, w825, w823) -> (resulting string=w810:string)  [unwired: 2 in, 1 out]
            "resulting string 2" <- w810
            n686 = String Subset(string=w810, offset (0)=0, length (rest)=4 ("length (rest)")) -> (substring=w805:string)
            n687 = String Subset(string=w810, offset (0)=4, length (rest)=4 ("length (rest)")) -> (substring=w840:string)
            n688 = String Subset(string=w810, offset (0)=8, length (rest)=4 ("length (rest)")) -> (substring=w839:string)
            n689 = String Subset(string=w810, offset (0)=12, length (rest)=4 ("length (rest)")) -> (substring=w818:string)
            n690 = String Subset(string=w810, offset (0)=16, length (rest)=4 ("length (rest)")) -> (substring=w816:string)
            n691 = Bundle(0, 0) -> (w799:cluster{i32, i32})  [unwired: 1 in]
            n692 = String Subset(string=w810, offset (0)=20, length (rest)=4 ("length (rest)")) -> (substring=w814:string)
            n693 = String Subset(string=w810, offset (0)=28, length (rest)=4 ("length (rest)")) -> (substring=w808:string)
            n694 = String Subset(string=w810, offset (0)=24, length (rest)=4 ("length (rest)")) -> (substring=w809:string)
            n695 = Hexadecimal String To Number(string=w805) -> (number=w822:u32)  [unwired: 2 in, 1 out]
            n696 = Hexadecimal String To Number(string=w840) -> (number=w821:u32)  [unwired: 2 in, 1 out]
            n697 = Hexadecimal String To Number(string=w839) -> (number=w838:u32)  [unwired: 2 in, 1 out]
            n698 = Hexadecimal String To Number(string=w818) -> (number=w837:u32)  [unwired: 2 in, 1 out]
            n699 = Hexadecimal String To Number(string=w816) -> (number=w815:u32)  [unwired: 2 in, 1 out]
            n700 = Hexadecimal String To Number(string=w814) -> (number=w813:u32)  [unwired: 2 in, 1 out]
            n701 = Hexadecimal String To Number(string=w809) -> (number=w807:u32)  [unwired: 2 in, 1 out]
            n702 = Hexadecimal String To Number(string=w808) -> (number=w806:u32)  [unwired: 2 in, 1 out]
            n703 = String To IP(1:"LAN Module IP Address") -> (0:w889:u32)
            n704 = Bundle("Voltage"=w798, "Phase"=w791) -> (w872:cluster{"Voltage ":dbl, "Phase ":dbl})  [unwired: 1 in]
            n705 = Compound Arithmetic op=ADD(w822, w821, w838, w837, w815, w813, w807, w806) -> (w834:u32)
            n706 = Build Array(w799, w872) -> (w873:cluster{"Voltage ":dbl, "Phase ":dbl}[])
            n707 = Number To Hexadecimal String(2:w834) -> (0:w833:string)  [unwired: 1 in]
            n708 = UDP Open(11:u16 40000 ("port")) -> (port=w886:refnum<k16>, 0:w885:errorcluster)  [unwired: 4 in, 1 out]
            n709 = String Subset(string=w833, offset (0)=1, length (rest)=4 ("length (rest)")) -> (substring=w832:string)
            n710 = Format Into String(format string="%01x%01x%06x%04x%04x%04x%04x%04x%04x%04s", "Data type", w831, w853, w794, w854, w830, w828, w826, w824, w832) -> (resulting string=w858:string)  [unwired: 2 in, 1 out]
            "Transmitted Data" <- w858
            n711 = String Length(string=w858) -> (length=w876:i32)
            n712 = Scale By Power Of 2(n=-1, x=w876) -> (x*2^n=w874:i32)
            n713 = for {
              N: w874 -> [_]
              shift-right: [w900] -> _
              shift-left: u32 0 -> [w901]
              tunnel: w858 -> [w899]
              tunnel: w879 -> [w898]
              tunnel: [w897] -> w878 mode=indexing
              tunnel: "%02x" ("format string") -> [w896]
              n714 = Scan From String(format string=w896, input string=w899, initial scan location=w901, default 1=w898) -> (offset past scan=w900:u32, output 1=w897:u8)  [unwired: 1 in, 2 out]
            }
            n715 = Type Cast(x=w878) -> (*(type *) &x=w857:string)  [unwired: 1 in]
            n716 = UDP Write(address=w889, port or service name="LAN Port", connection ID=w886, data in=w857, 8:w885) -> (error out=w888:errorcluster, 3:w887:refnum<k16>)  [unwired: 1 in]
            n717 = UDP Close(connection ID=w887, 8:w888) -> ()  [unwired: 2 out]
            n718 = property on="Phase 2" class="Pict"() -> ("Draw Area Size"=w871:T3)  [unwired: 2 in, 2 out]
            n719 = call <vilib>:"Polar Plot with Point Options.vi"("picture"=picture data[5B], "data array [mag, phase (deg)]"=w873, "dimensions (w,h)"=w871, "polar attributes"=T2 {"maximum"=0.0, "minimum"=0.0, "clip to min"=FALSE, "log?(F)"=FALSE, "grid color"=6710886, "plot color"=65280, "fmt and prec"={"format"=enum."Decimal", "precision"=2}, "visible section"=8}, "Lines/Points"=enum16{"Lines", "Points"}."Lines", "Size"=u16 5) -> ("new picture"=→"Phase 2":picture)  [unwired: 9 in]
          }
        }
      }
    }
    n720 = property on="Select test type" class="Ring (strict)"() -> ("RingText.Text"=w71:string)  [unwired: 2 in, 2 out]
    n721 = Wait (ms)(milliseconds to wait=u32 100) -> ()  [unwired: 1 out]
    n722 = TDMS Set Properties(5:w71, 7:"description", 8:w34, 11:w35) -> (0:w46:errorcluster, 3:w45:refnum<k34>)  [unwired: 2 in, 2 out]
    n723 = TDMS Set Properties(5:"s" ("channel name"), 7:"unit_string" ("channel name"), 8:w46, 9:"Time" ("channel name"), 10:w44, 11:w45) -> (0:w50:errorcluster, 3:w54:refnum<k34>)  [unwired: 2 out]
    n724 = local read "Phase unit"() -> (w33:u16)
    n725 = TDMS Set Properties(5:"volt" ("channel name"), 7:"unit_string" ("channel name"), 8:w50, 9:"Voltage" ("channel name"), 10:w44, 11:w54) -> (0:w49:errorcluster, 3:w53:refnum<k34>)  [unwired: 2 out]
    n726 = case shown="0, Default" w33 {
      tunnel: ["deg" ("channel name") "rad" ("channel name")] -> w32
      frame 0, Default {
      }
      frame 1 {
      }
    }
    n727 = TDMS Set Properties(5:w32, 7:"unit_string" ("channel name"), 8:w49, 9:"Phase" ("channel name"), 10:w44, 11:w53) -> (0:w48:errorcluster, 3:w52:refnum<k34>)  [unwired: 2 out]
    n728 = TDMS Set Properties(5:"Hz" ("channel name"), 7:"unit_string" ("channel name"), 8:w48, 9:"Frequency" ("channel name"), 10:w44, 11:w52) -> (0:w47:errorcluster, 3:w51:refnum<k34>)  [unwired: 2 out]
    n729 = TDMS Set Properties(5:"Hz/s" ("channel name"), 7:"unit_string" ("channel name"), 8:w47, 9:"ROCOF" ("channel name"), 10:w44, 11:w51) -> (0:w38:errorcluster, 3:w39:refnum<k34>)  [unwired: 2 out]
    n730 = Stop(stop? (T)="stop") -> ()
    "Numeric" <- w69
  }
  n731 = disable-structure shown="Enabled" {
    frame Disabled {
      n732 = while {
        stop <- w1046 stop-if-true
        w1046 = FALSE ("stop? (T)")
        n733 = event shown="[0] \"Voltage step\", \"Frequency step\", \"Start\": Value Change" {
          selector: _ -> [_ _]
          dyn-events: _ -> [_ _]
          timeout: _ -> [_ _]
          event "Voltage step", "Frequency step", "Start": Value Change {
            n734 = event-data() -> ()  [unwired: 1 in, 6 out]
            n735 = local write "Data type"(9 ("Data type")) -> ()
          }
          event "Start": Key Repeat {
            n736 = event-data() -> ()  [unwired: 1 in, 1 out]
          }
        }
        n737 = Stop(stop? (T)=w1046) -> ()
      }
    }
    frame Enabled {
    }
  }
  n738 = TDMS Close(8:w18, 11:w17) -> (0:w20:errorcluster, 3:w19:path)
  n739 = call <vilib>:"TDMS - File Viewer (NXG Style).vi"("error in"=w20, "file in"=w19) -> ("error out"=w21:errorcluster)  [unwired: 8 in, 1 out]
  n740 = call <vilib>:"Simple Error Handler.vi"("error in (no error)"=w21) -> ()  [unwired: 4 in, 5 out]
